vi "Imaging_Proc.vi"(5 "BioMAP file path":path=path "", 7 "Params.":variant, 8 "error in (no error)":errorcluster, 9 "Dynamic Params queue":refnum<queue>, 10 "Quit_UserEvent":refnum<user-event>, 11 "ControlQueueRef":variant) -> (0 "error out":errorcluster, 2 "Output":variant)   [LabVIEW 2013]
uses:
  Apps_static/ScanParams_SingleLine.ctl
  Files/BinaryHeader.ctl
  ControlDef/QueueRefs.ctl
  ControlDef/LaserCtrl_Method.ctl
  ControlDef/States-AToF.ctl
  <instrlib>/AnalogDiscSDKLv/VIs/DWF_CtrlQueue.ctl
  <instrlib>/AnalogDiscSDKLv/VIs/DWF_State.ctl
  <instrlib>/ESP300/Public/Data/ESP300_State.ctl
  <instrlib>/DG535/Command/DG535_States.ctl
  Hardware/BNC(QuantumComposers)/BNC_States.ctl
  Hardware/FemtoLaser(Legacy)/Laser_Status.ctl
  Hardware/DAQmx(Legacy)/DAQmx_Status.ctl
  ControlDef/Signal.ctl
  ProcessMethods/SignalAverager/ProcessStates.ctl
  Files/WriterState.ctl
  Files/Signal_Segment.ctl
  ControlDef/ProcessingMode.ctl
  Hardware/EPM2000(Legacy)/EPM2K_Status.ctl
  <instrlib>/AnalogDiscSDKLv/VIs/DWF_Signal.ctl
  ControlDef/SampleRateSelector.ctl
  DirectImaging_State.ctl
  Imaging_Params.ctl
  ProcessMethods/BioMapConversion/BioMAPWriterCoreParams.ctl
  <vilib>/Utility/miscctls.llb/LVRowAndColumnTypeDef.ctl
  <vilib>/picture/picture.llb/imagedata.ctl
  <userlib>/_OpenG.lib/comparison/comparison.llb/I32 Changed__ogtk.vi
  <vilib>/regexp/Match Regular Expression.xnode
  <instrlib>/ESP300/ESP300.lvlib
  <instrlib>/DG535/SRS_DG535_Lib.lvlib
  <userlib>/Utility/ErrorLog_lib.lvlib
  <instrlib>/AnalogDiscSDKLv/AnalogDiscSDKLv.lvlib
panel:
  in  "SaveImage":bool
  in  "Color Scheme":T1(ring)=enum."Rainbow"
  out "#SOL":i32
  out "#EOL":i32
  out "remaining lines":i32
  out "State":T2(ring)
  out "mzCali.":dbl[](array[numeric])
  out "Line#":i32
  in  "Cancel":bool
  in  "Close/Quit":bool
  in  "Peaks of Interest":string[][](table)=[["300", "300"], ["68", ".45"], ["92", ".45"], ["114", ".45"]]
  in  "conv. coeff.":sgl=6553.0
  out "# average":i32
  in  "Start":bool
  out "Intensity Graph":dbl[][](graph)
  in  "PeakOI #":i32
  out "MS (Raw)":cluster{"m/z_Array":dbl[], sgl[]}(graph)
  out "Iteration":i32
  out "Export File Path":path caption="Filename"
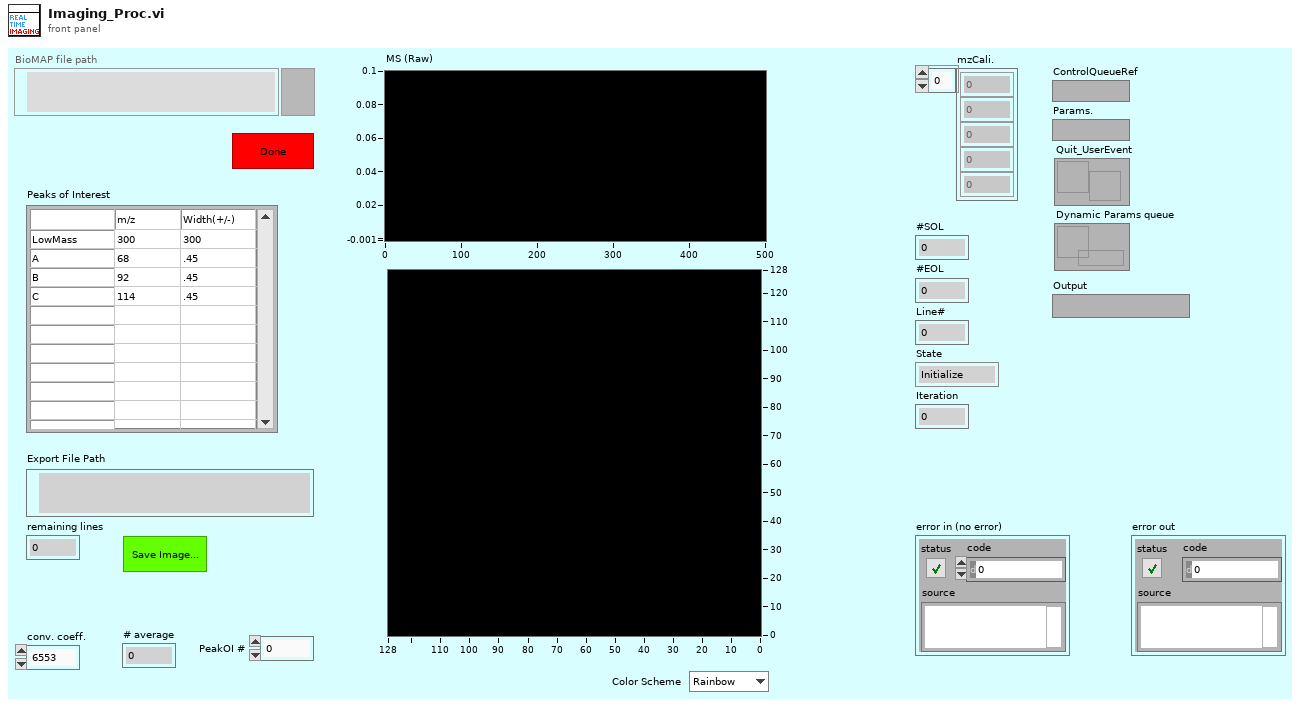
[diagram p1: front panel]
types:
  T1 = enum16{"Greyscale", "Rainbow", "Jet", "Rainbow_Wh", "Banded", "Seis", "InvertSeis", "Jaisnd", "TBD1"}
  T2 = enum16{"Initialize", "Open", "PrepScanParams", "WaitData", "Flush", "ScanResult", "CheckEndCondition", "Close", "Quit", "Refresh_Image", "Refresh_Profile", "Refresh_Spectra", "Refresh_RawSpectrum", "SaveMiddleFile"}
  T3 = enum8{"Enabled", "Disabled", "Disabled and Grayed Out"}
  T4 = typedef "QueueRefs.ctl" = cluster{"LaserCtrlMethod":T5, "Apps":refnum<queue>, "MainDAQCoreQueue":refnum<queue>, "Micos":refnum<queue>, "ESP300":refnum<queue>, "SMC100":refnum<queue>, "SRS DG535":refnum<queue>, "BNC":refnum<queue>, "SDG_ii":refnum<queue>, "NI-USB_DAQmx":refnum<queue>, "ProcCore_CtrlQueue":refnum<queue>, "WriterCtrl":refnum<queue>, "WriterSIG":refnum<queue>, "Feedback":refnum<queue>, "EPM2000":refnum<queue>, "InfoRef":refnum<vi>, "AppsLock":T6, "ProcCore_SignalQueue":refnum<queue>}
  T5 = typedef "LaserCtrl_Method.ctl" = enum16{"SRS_DG535", "BNC", "SDG_II"}
  T6 = typedef "Semaphore RefNum" = refnum<k1>
  T7 = typedef "ProcessStates.ctl" = enum16{"Initialize", "Normal", "Display", "Write2Buffer", "CalcMzArray", "StartSave", "StopSave", "ConfigChanged", "EndOfLine", "SetFilterParams", "SetGraphsEnable", "SetAcquisitionParams", "ChangeDisplayIncrement", "ChangeRepRate", "SetWriterRef", "Quit", "StartOfLine"}
  T8 = cluster{"Average":i32, "X (Img)":i32, "Y (Img)":i32, "Spectra":sgl[], "Depth":i32}
  T9 = typedef "BioMAPWriterCoreParams.ctl" = cluster{"File Header":T10, "mzCali.":dbl[], "m/z_Array":dbl[], "SampleRate":T11, "TrigDelay":dbl, "file refnum":refnum<file>, "file path":path, "PeakOI":cluster{"m/z":dbl, "Width(+/-)":dbl}[]}
  T10 = typedef "BinaryHeader.ctl" = cluster{"Start Position":dbl[], "StepWidth":dbl[], "Dimension":i32[], "SpecLength":i32}
  T11 = typedef "SampleRateSelector.ctl" = dbl
  T12 = typedef "Imaging_Params.ctl" = cluster{"File Header":T10, "ScanSpeed":dbl, "HighSpeed":dbl, "SampleRate":T11, "Rep.Rate (Hz)":dbl, "TrigDelay":dbl, "mzCali":dbl[], "KeepStill(ms)":u32, "SaveRaw":bool}
  T13 = typedef "DirectImaging_State.ctl" = cluster{"State":enum16{"Initialize", "Open", "PrepScanParams", "WaitData", "Flush", "ScanResult", "CheckEndCondition", "Close", "Quit", "Refresh_Image", "Refresh_Profile", "Refresh_Spectra", "Refresh_RawSpectrum", "SaveMiddleFile", "Save_Image"}, "Para.":variant}
  T14 = cluster{"Save?":bool, "File Header":T10, "Scan#":i32, "ControlRefs":T4, "HighSpeed":dbl, "ScanSpeed":dbl, "SampleRate":T11, "mzCali.":dbl[], "TrigDelay":dbl}
  T15 = typedef "LVRowAndColumnTypeDef.ctl" = cluster{"Row":i32, "Column":i32}
  T16 = cluster{"queue out":refnum<queue>, "queue out":refnum<queue>}
  T17 = typedef "Signal.ctl" = cluster{"Command":T7, "Params":variant}
  T18 = typedef "Signal_Segment.ctl" = cluster{"SampleRate":dbl, "TrigDelay":dbl, "SpecLength":dbl, "DAQ_Range":dbl, "Average#":i32, "Position":dbl[], "Spectrum":sgl[], "Calibr.":dbl[], "Pressure":dbl, "Desp_LaserEnergy":dbl, "PI_LaserEnergy":dbl, "Voltages Table":sgl[][], "ProcMode":T19, "Threshold":dbl, "Comment":string, "TickCount":dbl, "Time Stamp":timestamp}
  T19 = typedef "ProcessingMode.ctl" = enum16{"None", "Drop by Threshold", "TDC Simulate", "SetFilter"}
  T20 = enum16{"open", "replace", "create", "open or create", "replace or create", "replace or create with confirmation"}
  T21 = typedef "ScanParams_SingleLine.ctl" = cluster{"Start Position":dbl[], "End Position":dbl[], "HighSpeed":dbl, "ScanSpeed":dbl, "KeepStill(ms)":u32}
  T22 = cluster{"Dimension":u16, "SpecDepth":u16, "x dimension":u16, "y dimension":u16, "z dimension":u16}
  T23 = cluster{"Dimension 1":sgl, "Dimension 2":sgl, "Dimension 3":sgl, "Dimension 4":sgl, "Dimension 5":sgl, "Dimension 6":sgl, "Dimension 7":sgl, "Dimension 8":sgl}
  T24 = typedef "imagedata.ctl" = cluster{"image type":i32, "image depth":i32, "image":u8[], "mask":u8[], "colors":u32[], "Rectangle":cluster{"left":i16, "top":i16, "right":i16, "bottom":i16}}
  T25 = cluster{"Rows Per Strip":i32, "Photometric":i32, "Compression Type":i32}
  T26 = enum16{"Initialize", "Open", "PrepScanParams", "WaitData", "Flush", "ScanResult", "CheckEndCondition", "Close", "Quit", "Refresh_Image", "Refresh_Profile", "Refresh_Spectra", "Refresh_RawSpectrum", "SaveMiddleFile", "Save_Image"}
  T27 = typedef "IMAQ Image.ctl" = refnum<image>
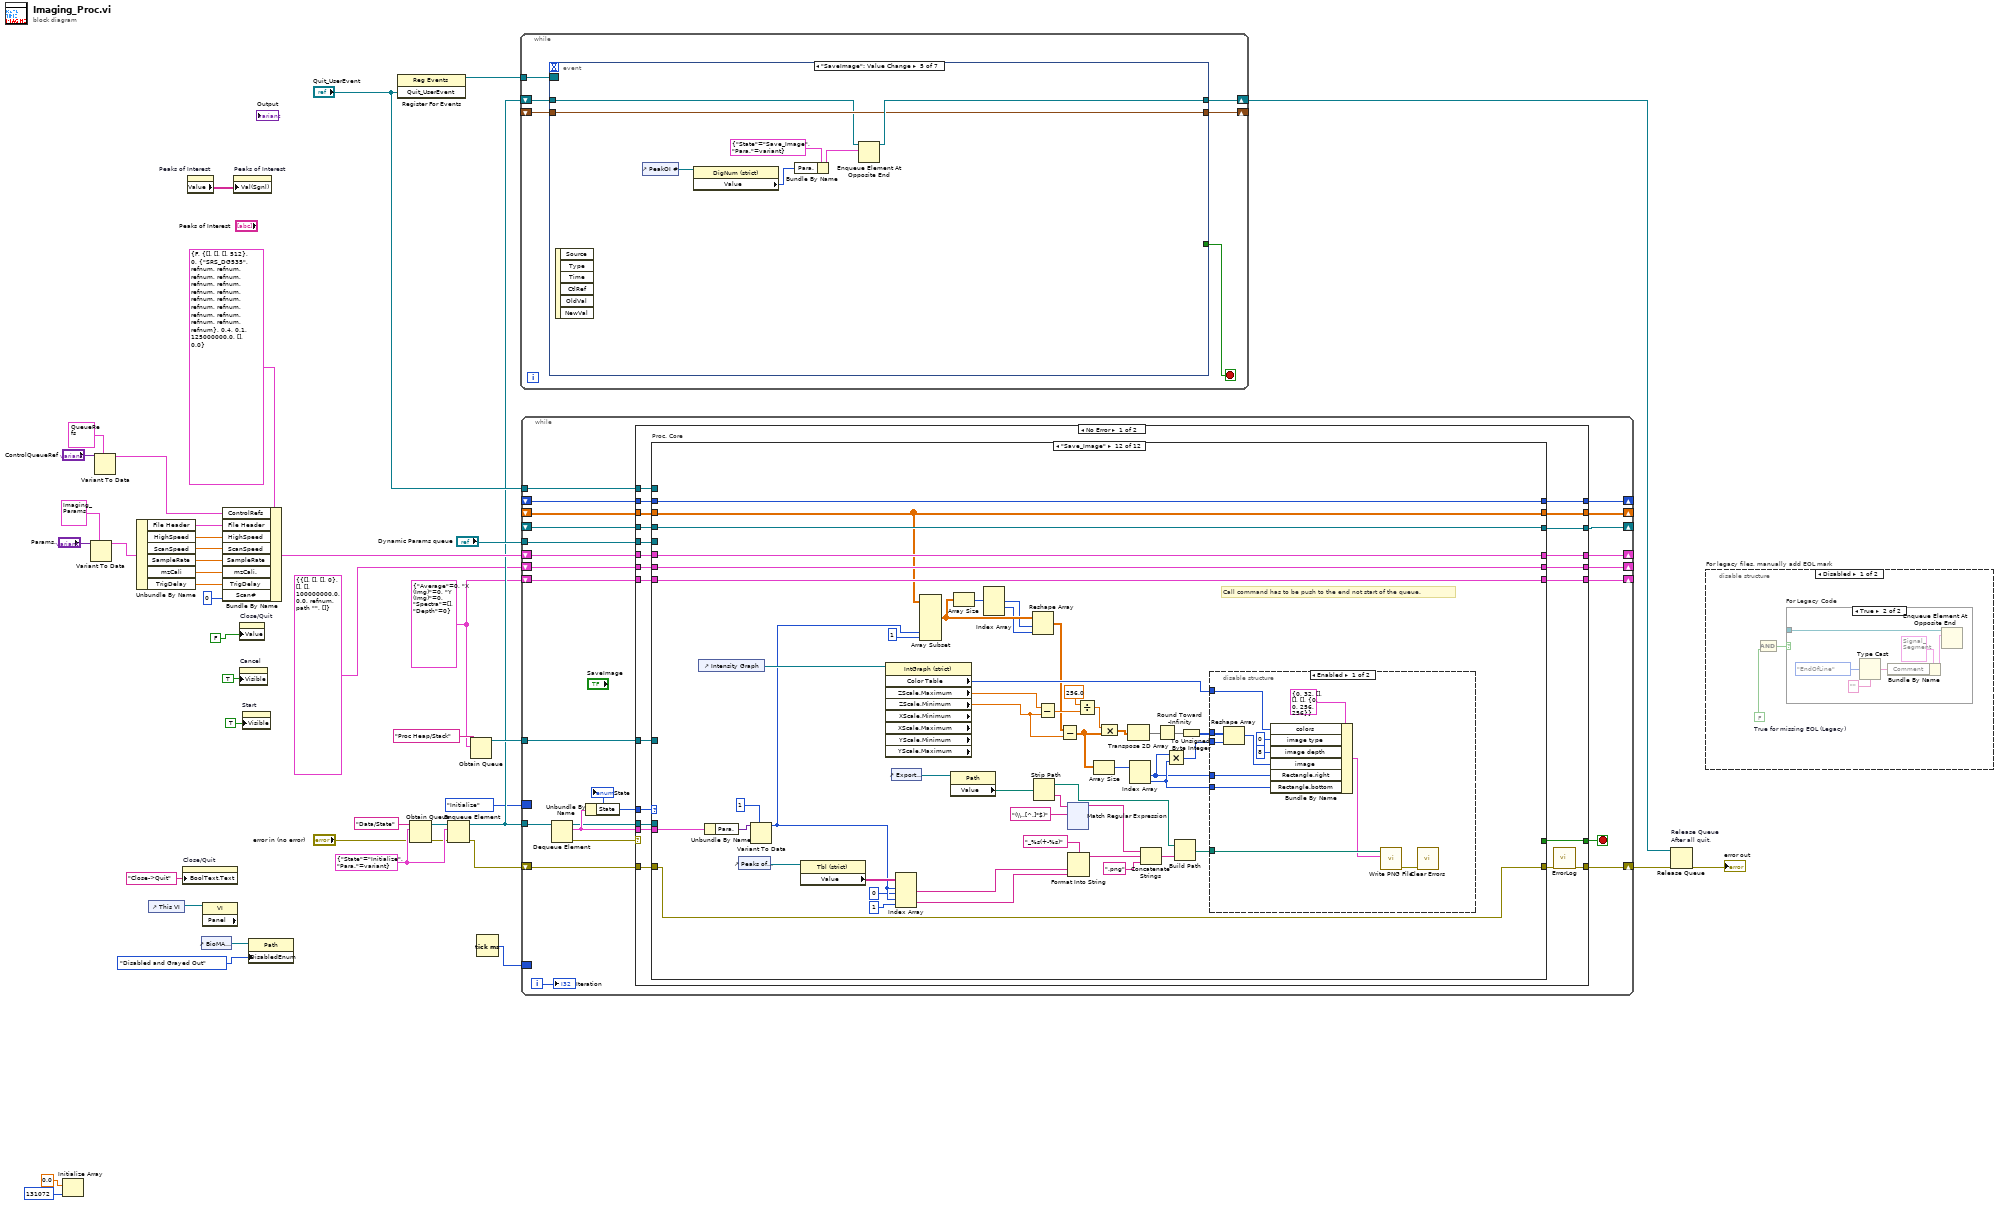
[diagram p0: block diagram]
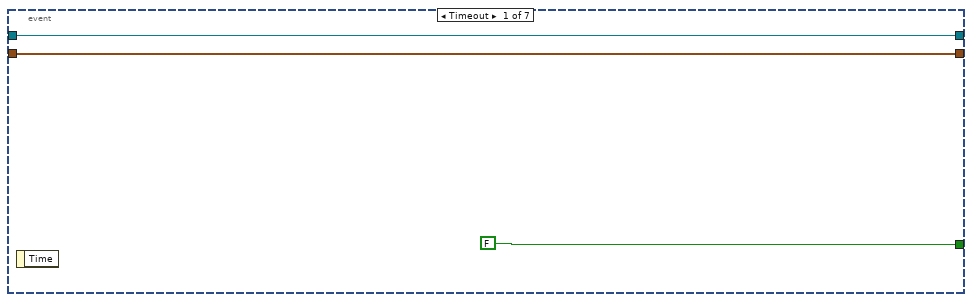
[diagram p4: hidden frame]
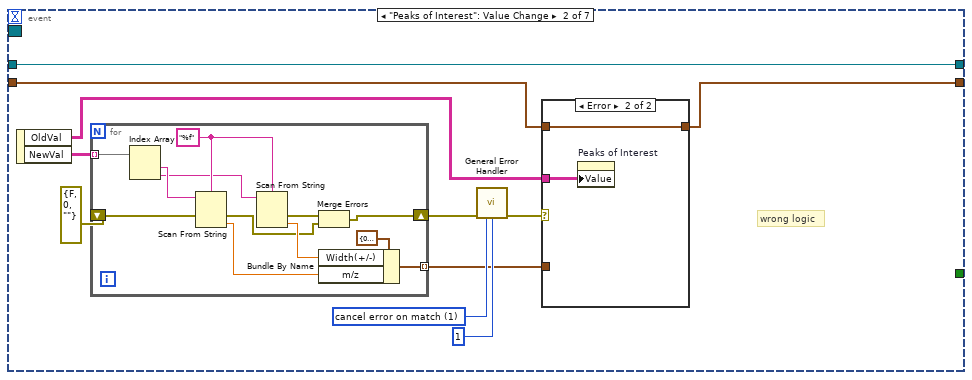
[diagram p5: hidden frame]
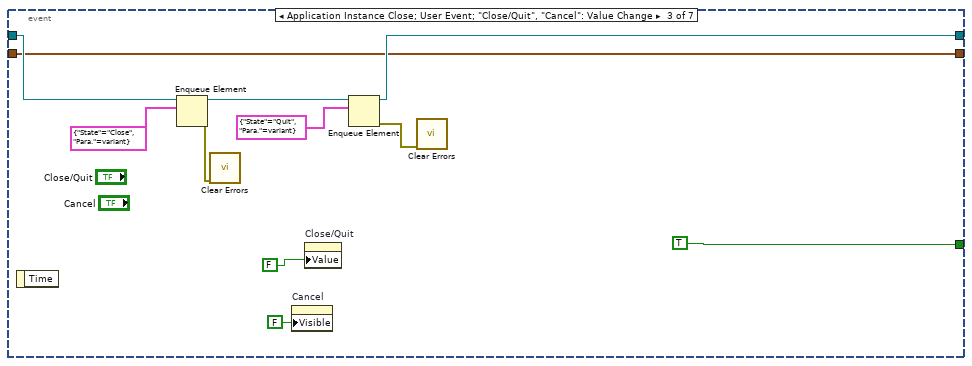
[diagram p7: hidden frame]
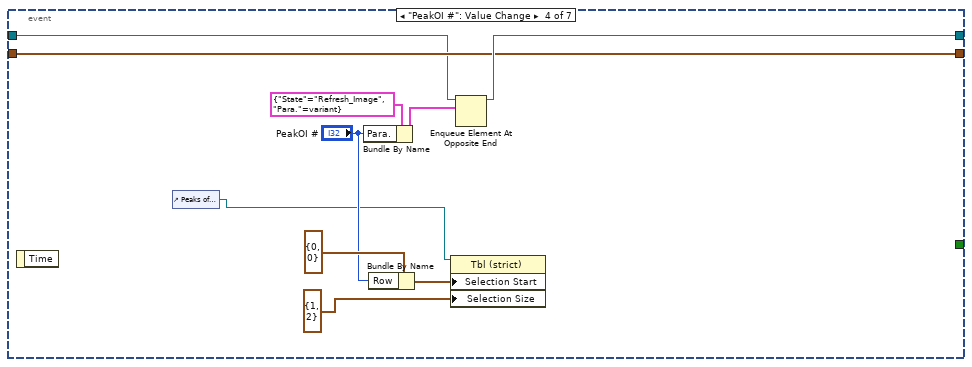
[diagram p8: hidden frame]
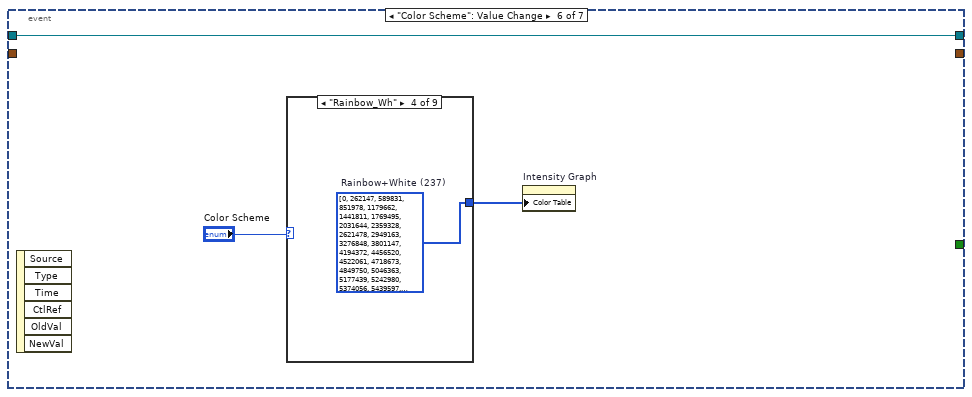
[diagram p9: hidden frame]
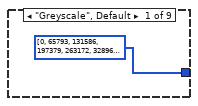
[diagram p10: hidden frame]
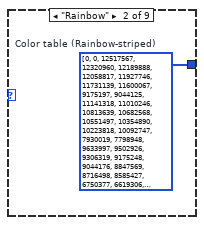
[diagram p11: hidden frame]
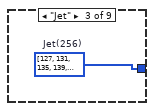
[diagram p12: hidden frame]
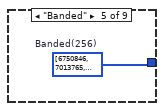
[diagram p13: hidden frame]
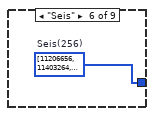
[diagram p14: hidden frame]
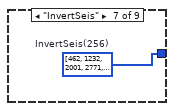
[diagram p15: hidden frame]
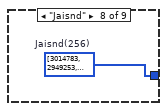
[diagram p16: hidden frame]
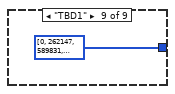
[diagram p17: hidden frame]
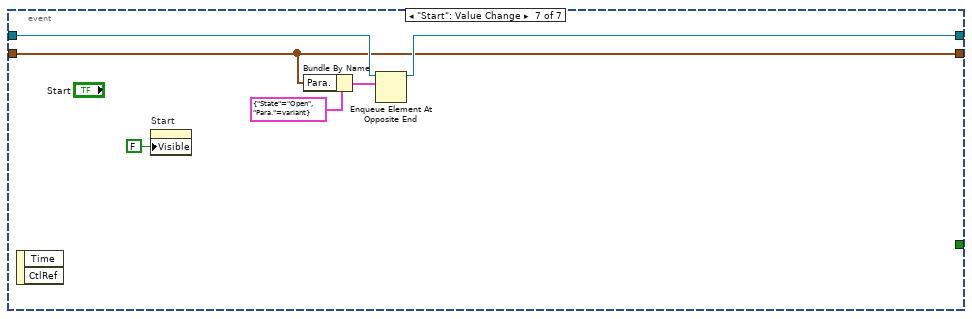
[diagram p18: hidden frame]
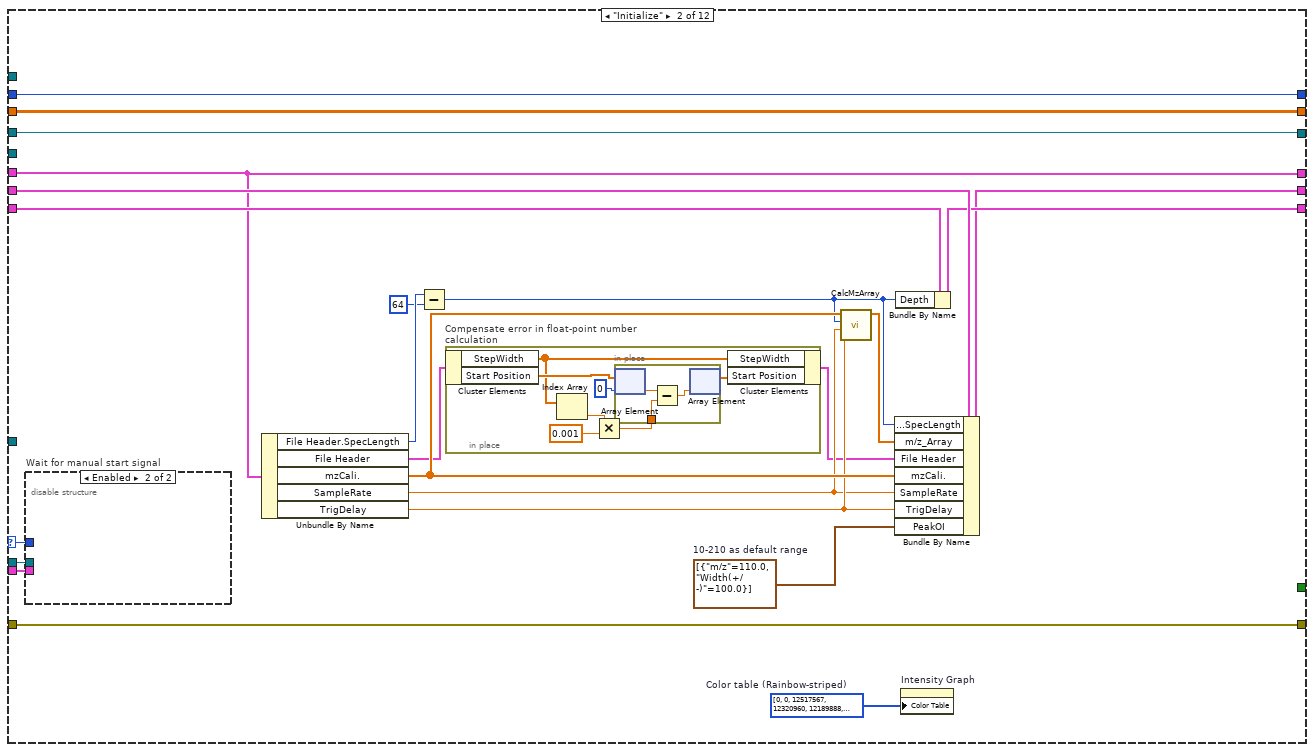
[diagram p20: hidden frame]
diagram:
  w22 = T8 {"Average"=0, "X (Img)"=0, "Y (Img)"=0, "Spectra"=[], "Depth"=0} ("output cluster")
  w34 = T13 {"State"=enum."Initialize", "Para."=variant}
  n1 = Initialize Array(sgl 0.0 ("element"), 131072 ("dimension size")) -> ()  [unwired: 1 out]
  n2 = Variant To Data(type=T12 {"File Header"={"Start Position"=[], "StepWidth"=[], "Dimension"=[], "SpecLength"=0}, "ScanSpeed"=0.0, "HighSpeed"=0.0, "SampleRate"=0.0, "Rep.Rate (Hz)"=0.0, "TrigDelay"=0.0, "mzCali"=[], "KeepStill(ms)"=0, "SaveRaw"=FALSE} ("BeamProfiling_Params"), Variant="Params.") -> (data=w29:T12)  [unwired: 1 in, 1 out]
  n3 = Variant To Data(type=T4 {"LaserCtrlMethod"=enum."SRS_DG535", "Apps"=refnum, "MainDAQCoreQueue"=refnum, "Micos"=refnum, "ESP300"=refnum, "SMC100"=refnum, "SRS DG535"=refnum, "BNC"=refnum, "SDG_ii"=refnum, "NI-USB_DAQmx"=refnum, "ProcCore_CtrlQueue"=refnum, "WriterCtrl"=refnum, "WriterSIG"=refnum, "Feedback"=refnum, "EPM2000"=refnum, "InfoRef"=refnum, "AppsLock"=refnum, "ProcCore_SignalQueue"=refnum} ("ControlRefs"), Variant="ControlQueueRef") -> (data=w8:T4)  [unwired: 1 in, 1 out]
  n4 = Unbundle By Name(w29) -> ("File Header"=w28:T10, "HighSpeed"=w27:dbl, "ScanSpeed"=w26:dbl, "SampleRate"=w24:T11, "mzCali"=w14:dbl[], "TrigDelay"=w13:dbl)
  n5 = control-ref of="This VI"() -> (w12:refnum<vi>)
  n6 = property on="Close/Quit" class="Bool (strict)"("BoolText.Text"="Close->Quit" ("Boolean Text.Text")) -> ()  [unwired: 2 in, 2 out]
  n7 = property on="Peaks of Interest" class="Tbl (strict)"() -> ("Value"=w2:string[][])  [unwired: 2 in, 2 out]
  n8 = control-ref of="BioMAP file path"() -> (w7:refnum<vi>)
  n9 = property class="VI" props=["Panel"](reference=w12) -> ()  [unwired: 1 in, 3 out]
  n10 = Bundle By Name(cluster=T14 {"Save?"=FALSE, "File Header"={"Start Position"=[], "StepWidth"=[], "Dimension"=[], "SpecLength"=512}, "Scan#"=0, "ControlRefs"={"LaserCtrlMethod"=enum."SRS_DG535", "Apps"=refnum, "MainDAQCoreQueue"=refnum, "Micos"=refnum, "ESP300"=refnum, "SMC100"=refnum, "SRS DG535"=refnum, "BNC"=refnum, "SDG_ii"=refnum, "NI-USB_DAQmx"=refnum, "ProcCore_CtrlQueue"=refnum, "WriterCtrl"=refnum, "WriterSIG"=refnum, "Feedback"=refnum, "EPM2000"=refnum, "InfoRef"=refnum, "AppsLock"=refnum, "ProcCore_SignalQueue"=refnum}, "HighSpeed"=0.4, "ScanSpeed"=0.1, "SampleRate"=125000000.0, "mzCali."=[], "TrigDelay"=0.0} ("output cluster"), "ControlRefs"=w8, "File Header"=w28, "HighSpeed"=w27, "ScanSpeed"=w26, "SampleRate"=w24, "mzCali."=w14, "TrigDelay"=w13, "Scan#"=0) -> (w38:T14)
  n11 = property on="Peaks of Interest" class="Tbl (strict)"("Val(Sgnl)"=w2) -> ()  [unwired: 2 in, 2 out]
  n12 = property on="Close/Quit" class="Bool (strict)"("Value"=FALSE) -> ()  [unwired: 2 in, 2 out]
  n13 = property on="Cancel" class="Bool"("Visible"=TRUE) -> ()  [unwired: 2 in, 2 out]
  n14 = property on="Start" class="Bool"("Visible"=TRUE) -> ()  [unwired: 2 in, 2 out]
  n15 = property class="Path"(reference=w7, "DisabledEnum"=T3."Disabled and Grayed Out" ("Disabled")) -> ()  [unwired: 1 in, 2 out]
  n16 = register-events("Quit_UserEvent") -> (reference out=w39:refnum<event-registration>)  [unwired: 2 in, 1 out]
  n17 = Obtain Queue(name (unnamed)="Data/State", element data type=w34, error in (no error)="error in (no error)") -> (queue out=w35:refnum<queue>, error out=w33:errorcluster)  [unwired: 2 in, 1 out]
  n18 = Enqueue Element(queue=w35, element=w34, error in (no error)=w33) -> (queue out=w31:refnum<queue>, error out=w23:errorcluster)  [unwired: 1 in, 1 out]
  n19 = Obtain Queue(name (unnamed)="Proc Heap/Stack", element data type=w22) -> (queue out=w44:refnum<queue>)  [unwired: 3 in, 2 out]
  n20 = Tick Count (ms)() -> (millisecond timer value=w21:u32)
  n21 = while {
    tunnel: w39 -> [w48]
    shift-right: [w47] -> w15
    shift-left: w31 -> [w50]
    shift-right: [w46] -> _
    shift-left: _ -> [w45]
    stop <- w49 stop-if-true
    n22 = event shown="[4] \"SaveImage\": Value Change" {
      selector: w48 -> [_ _ _ _ _ _ _]
      dyn-events: _ -> [_ _ _ _ _ _ _]
      timeout: _ -> [_ _ _ _ _ _ _]
      tunnel: w50 -> [w52 w62 w87 w96 w103 w110 w125]
      tunnel: [FALSE _ TRUE _ _ _ _] -> w49
      tunnel: [w52 w62 w83 w98 w105 w110 w123] -> w47
      tunnel: [w51 w56 w82 w97 w104 _ w121] -> w46
      tunnel: w45 -> [w51 w54 w82 w97 w104 _ w121]
      event Timeout {
        n23 = event-data() -> ()  [unwired: 1 in, 1 out]
      }
      event "Peaks of Interest": Value Change {
        w57 = 1 items=["no exception", "cancel error on match", "set error on match"] ("[exception action] (none:0)")
        # "wrong logic"
        n24 = event-data() -> ("OldVal"=w63:string[][], "NewVal"=w64:string[][])  [unwired: 1 in]
        n25 = for {
          tunnel: w64 -> [w76] mode=indexing
          shift-right: [w68] -> w58
          shift-left: errorcluster {"status"=FALSE, "code"=0, "source"=""} ("error IO") -> [w70]
          tunnel: [w69] -> w55 mode=indexing
          w75 = "%f" ("format string")
          n26 = Index Array(array=w76) -> (element #1=w66:string, element #2=w65:string)  [unwired: 2 in]
          n27 = Scan From String(format string=w75, input string=w66, error in=w70) -> (error out=w67:errorcluster, output 1=w72:dbl)  [unwired: 2 in, 2 out]
          n28 = Scan From String(format string=w75, input string=w65) -> (error out=w71:errorcluster, output 1=w73:dbl)  [unwired: 3 in, 2 out]
          n29 = Merge Errors(w71, w67) -> (w68:errorcluster)
          n30 = Bundle By Name(cluster=cluster{"m/z":dbl, "Width(+/-)":dbl} {"m/z"=0.0, "Width(+/-)"=0.0} ("Peak-Of-Interest"), "Width(+/-)"=w73, "m/z"=w72) -> (w69:cluster{"m/z":dbl, "Width(+/-)":dbl})
        }
        n31 = call <vilib>:"General Error Handler.vi"("error in (no error)"=w58, "[exception action] (none:0)"=w57, "[exception code]"=1) -> ("error out"=w59:errorcluster)  [unwired: 8 in, 4 out]
        n32 = case shown="Error" w59 {
          tunnel: w63 -> [_ w79]
          tunnel: [w77 w78] -> w56
          tunnel: w55 -> [w77 _]
          tunnel: w54 -> [_ w78]
          frame No Error {
          }
          frame Error {
            n33 = property on="Peaks of Interest" class="Tbl (strict)"("Value"=w79) -> ()  [unwired: 2 in, 2 out]
          }
        }
      }
      event Application Instance Close; User Event; "Close/Quit", "Cancel": Value Change {
        n34 = event-data() -> ()  [unwired: 1 in, 1 out]
        n35 = Enqueue Element(queue=w87, element=T13 {"State"=enum."Close", "Para."=variant}) -> (queue out=w88:refnum<queue>, error out=w86:errorcluster)  [unwired: 2 in, 1 out]
        n36 = call <vilib>:"Clear Errors.vi"("error in (no error)"=w86) -> ()  [unwired: 6 in, 1 out]
        n37 = property on="Cancel" class="Bool"("Visible"=FALSE) -> ()  [unwired: 2 in, 2 out]
        n38 = property on="Close/Quit" class="Bool (strict)"("Value"=FALSE) -> ()  [unwired: 2 in, 2 out]
        n39 = Enqueue Element(queue=w88, element=T13 {"State"=enum."Quit", "Para."=variant}) -> (queue out=w83:refnum<queue>, error out=w89:errorcluster)  [unwired: 2 in, 1 out]
        n40 = call <vilib>:"Clear Errors.vi"("error in (no error)"=w89) -> ()  [unwired: 6 in, 1 out]
      }
      event "PeakOI #": Value Change {
        n41 = event-data() -> ()  [unwired: 1 in, 1 out]
        n42 = control-ref of="Peaks of Interest"() -> (w91:refnum<vi>)
        n43 = Bundle By Name(cluster=T13 {"State"=enum."Refresh_Image", "Para."=variant} ("element"), "Para."="PeakOI #") -> (w99:T13)
        n44 = Bundle By Name(cluster=T15 {"Row"=0, "Column"=0} ("Selection Start"), "Row"="PeakOI #") -> (w94:T15)
        n45 = property on="Property Node" class="Tbl (strict)"(reference=w91, "Selection Start"=w94, "Selection Size"=T15 {"Row"=1, "Column"=2}) -> ()  [unwired: 1 in, 2 out]
        n46 = Enqueue Element At Opposite End(queue=w96, element=w99) -> (queue out=w98:refnum<queue>)  [unwired: 2 in, 2 out]
      }
      event "SaveImage": Value Change {
        n47 = event-data() -> ()  [unwired: 1 in, 6 out]
        n48 = control-ref of="PeakOI #"() -> (w102:refnum<vi>)
        n49 = property class="DigNum (strict)"(reference=w102) -> ("Value"=w101:i32)  [unwired: 1 in, 2 out]
        n50 = Bundle By Name(cluster=T13 {"State"=enum."Save_Image", "Para."=variant} ("element"), "Para."=w101) -> (w106:T13)
        n51 = Enqueue Element At Opposite End(queue=w103, element=w106) -> (queue out=w105:refnum<queue>)  [unwired: 2 in, 2 out]
      }
      event "Color Scheme": Value Change {
        n52 = event-data() -> ()  [unwired: 1 in, 6 out]
        n53 = case shown="\"Rainbow_Wh\"" "Color Scheme" {
          tunnel: [u32[] [0, 65793, 131586, 197379, 263172, 328965, 394758, 460551, 526344, 592137, 657930, 723723, 789516, 855309, 921102, 986895, 1052688, 1118481, 1184274, 1250067, 1315860, 1381653, 1447446, 1513239, 1579032, 1644825, 1710618, 1776411, 1842204, 1907997, 1973790, 2039583, 2105376, 2171169, 2236962, 2302755, 2368548, 2434341, 2500134, 2565927, 2631720, 2697513, 2763306, 2829099, 2894892, 2960685, 3026478, 3092271, 3158064, 3223857, 3289650, 3355443, 3421236, 3487029, 3552822, 3618615, 3684408, 3750201, 3815994, 3881787, 3947580, 4013373, 4079166, 4144959, 4210752, 4276545, 4342338, 4408131, 4473924, 4539717, 4605510, 4671303, 4737096, 4802889, 4868682, 4934475, 5000268, 5066061, 5131854, 5197647, 5263440, 5329233, 5395026, 5460819, 5526612, 5592405, 5658198, 5723991, 5789784, 5855577, 5921370, 5987163, 6052956, 6118749, 6184542, 6250335, 6316128, 6381921, 6447714, 6513507, 6579300, 6645093, 6710886, 6776679, 6842472, 6908265, 6974058, 7039851, 7105644, 7171437, 7237230, 7303023, 7368816, 7434609, 7500402, 7566195, 7631988, 7697781, 7763574, 7829367, 7895160, 7960953, 8026746, 8092539, 8158332, 8224125, 8289918, 8355711, 8421504, 8487297, 8553090, 8618883, 8684676, 8750469, 8816262, 8882055, 8947848, 9013641, 9079434, 9145227, 9211020, 9276813, 9342606, 9408399, 9474192, 9539985, 9605778, 9671571, 9737364, 9803157, 9868950, 9934743, 10000536, 10066329, 10132122, 10197915, 10263708, 10329501, 10395294, 10461087, 10526880, 10592673, 10658466, 10724259, 10790052, 10855845, 10921638, 10987431, 11053224, 11119017, 11184810, 11250603, 11316396, 11382189, 11447982, 11513775, 11579568, 11645361, 11711154, 11776947, 11842740, 11908533, 11974326, 12040119, 12105912, 12171705, 12237498, 12303291, 12369084, 12434877, 12500670, 12566463, 12632256, 12698049, 12763842, 12829635, 12895428, 12961221, 13027014, 13092807, 13158600, 13224393, 13290186, 13355979, 13421772, 13487565, 13553358, 13619151, 13684944, 13750737, 13816530, 13882323, 13948116, 14013909, 14079702, 14145495, 14211288, 14277081, 14342874, 14408667, 14474460, 14540253, 14606046, 14671839, 14737632, 14803425, 14869218, 14935011, 15000804, 15066597, 15132390, 15198183, 15263976, 15329769, 15395562, 15461355, 15527148, 15592941, 15658734, 15724527, 15790320, 15856113, 15921906, 15987699, 16053492, 16119285, 16185078, 16250871, 16316664, 16382457, 16448250, 16514043, 16579836, 16645629, 16711422, 16777215] ("Array") w112 w113 w114 w115 w116 w117 w118 u32[] [0, 262147, 589831, 851978, 1179662, 1441811, 1769495, 2031644, 2359328, 2621478, 2949163, 3276848, 3801147, 4194372, 4456520, 4522061, 4718673, 4849750, 5046363, 5177439, 5242980, 5374056, 5439597, 5505142, 5636218, 5767300, 5636232, 5701773, 5701777, 5701782, 5570714, 5505183, 5505187, 5505192, 5177521, 5111990, 5046458, 4980927, 4587720, 4456652, 4325585, 3932374, 3801306, 3604703, 3014888, 2818284, 2621681, 2359541, 2162938, 1638655, 1048831, 786687, 262399, 255, 1279, 4351, 5631, 6655, 7679, 9983, 11007, 12031, 13311, 16383, 17407, 18687, 21759, 23039, 24063, 25087, 27391, 28415, 29439, 30719, 32767, 34815, 36095, 39167, 40447, 41471, 42495, 44799, 45823, 46847, 48127, 50175, 51199, 55551, 56575, 57855, 58879, 59903, 62207, 63231, 64255, 65535, 65526, 65522, 65518, 65505, 65496, 65492, 65483, 65479, 65475, 65471, 65467, 65458, 65454, 65450, 65437, 65432, 65424, 65415, 65411, 65407, 65403, 65394, 65390, 65386, 65382, 65369, 65364, 65360, 65356, 65343, 65339, 65335, 65326, 65322, 65318, 65305, 65301, 65296, 65292, 65288, 65280, 589568, 851712, 1441536, 1703680, 1965824, 2817792, 3079936, 3407616, 3669760, 4194048, 4456192, 4783872, 5046016, 5897984, 6160128, 6422272, 7274240, 7536384, 7864064, 8126208, 8650496, 8912640, 9240320, 9502464, 10092288, 10616576, 10878720, 11730688, 11992832, 12320512, 12582656, 13106944, 13369088, 13696768, 13958912, 14548736, 14810880, 15924992, 16187136, 16449280, 16776960, 16775680, 16773632, 16772608, 16771328, 16770304, 16768256, 16766976, 16765952, 16762624, 16760576, 16759552, 16757248, 16756224, 16755200, 16753920, 16752896, 16750848, 16749568, 16748544, 16745216, 16744192, 16742144, 16739840, 16738816, 16737792, 16736512, 16734464, 16733440, 16732160, 16731136, 16727808, 16726784, 16725760, 16724736, 16721408, 16720384, 16719104, 16717056, 16716032, 16714752, 16711680, 16711680, 16711680, 16711680, 16711680, 16711680, 16711680, 16711680, 16711680, 16711680, 16711680, 16711680, 16711680, 16711680, 16711680, 16711680, 16711680, 16711680, 15527148, 15592941, 15658734, 15724527, 15790320, 15856113, 15921906, 15987699, 16053492, 16119285, 16185078, 16250871, 16316664, 16382457, 16448250, 16514043, 16579836, 16645629, 16711422, 16777215] ("appended array")] -> w108
          frame "Greyscale", Default {
          }
          frame "Rainbow" {
            w112 = u32[] [0, 0, 12517567, 12320960, 12189888, 12058817, 11927746, 11731139, 11600067, 9175197, 9044125, 11141318, 11010246, 10813639, 10682568, 10551497, 10354890, 10223818, 10092747, 7930019, 7798948, 9633997, 9502926, 9306319, 9175248, 9044176, 8847569, 8716498, 8585427, 6750377, 6619306, 8126677, 7995606, 7798999, 7667927, 7536856, 7340249, 7209178, 7078106, 5505199, 5374128, 6619357, 6488285, 6291678, 6160607, 6029536, 5832929, 5701857, 5570786, 4325557, 4194486, 5112036, 4980965, 4784358, 4653287, 4522215, 4325608, 4194537, 4063466, 3080380, 3014844, 3604716, 3408109, 3277038, 3277038, 3145966, 3014895, 2818288, 2687217, 2556145, 1900738, 1769666, 2097396, 1900789, 1769717, 1638646, 1507575, 1310968, 1179896, 1048825, 721096, 590024, 590075, 393468, 262397, 131326, 255, 1791, 3327, 4863, 5068, 6348, 9471, 11007, 12543, 14079, 15615, 17151, 18687, 20223, 17612, 18636, 25087, 26623, 28159, 29695, 31231, 32767, 34303, 35839, 29900, 31180, 40447, 41983, 43775, 45311, 46847, 48383, 49919, 51455, 42444, 43724, 56063, 57599, 59135, 60671, 62207, 63743, 65535, 65528, 52418, 52413, 65510, 65504, 65498, 65492, 65486, 65480, 65474, 65468, 52369, 52364, 65449, 65443, 65437, 65431, 65425, 65419, 65413, 65407, 52321, 52316, 65389, 65383, 65377, 65371, 65364, 65358, 65352, 65346, 52272, 52267, 65328, 65322, 65316, 65310, 65304, 65298, 65292, 65286, 52224, 314368, 851712, 1244928, 1638144, 2031360, 2424576, 2817792, 3211008, 3604224, 3197952, 3525632, 4783872, 5177088, 5635840, 6029056, 6422272, 6815488, 7208704, 7601920, 6409216, 6736896, 6736896, 8781568, 9174784, 9568000, 9961216, 10354432, 10747648, 11206400, 11599616, 9554944, 9882624, 12779264, 13172480, 13565696, 13958912, 14352128, 14745344, 15138560, 15531776, 12766208, 13093888, 16776960, 16775170, 16773637, 16771847, 16770314, 16768780, 16766991, 16765457, 13411088, 13409810, 16760601, 16758812, 16757278, 16755745, 16753955, 16752422, 16750888, 16749099, 13398052, 13396774, 16744243, 16742704, 16741166, 16739884, 16738345, 16736807, 16735269, 16733730, 13385753, 13384728, 16729371, 16727833, 16726295, 16725012, 16723474, 16721936, 16720397, 16718859, 13373959, 13372677, 16714500, 16712962, 16777215]  # Color table (Rainbow-striped)
          }
          frame "Jet" {
            w113 = u32[] [127, 131, 135, 139, 143, 147, 151, 155, 159, 163, 167, 171, 175, 179, 183, 187, 191, 195, 199, 203, 207, 211, 215, 219, 223, 227, 231, 235, 239, 243, 247, 251, 255, 1279, 2303, 3327, 4351, 5375, 6399, 7423, 8447, 9471, 10495, 11519, 12543, 13567, 14591, 15615, 16639, 17663, 18687, 19711, 20735, 21759, 22783, 23807, 24831, 25855, 26879, 27903, 28927, 29951, 30975, 31999, 33023, 34047, 35071, 36095, 37119, 38143, 39167, 40191, 41215, 42239, 43263, 44287, 45311, 46335, 47359, 48383, 49407, 50431, 51455, 52479, 53503, 54527, 55551, 56575, 57599, 58623, 59647, 60671, 61695, 62719, 63743, 64767, 131069, 393209, 655349, 917489, 1179629, 1441769, 1703909, 1966049, 2228189, 2490329, 2752469, 3014609, 3276749, 3538889, 3801029, 4063169, 4325309, 4587449, 4849589, 5111729, 5373869, 5636009, 5898149, 6160289, 6422429, 6684569, 6946709, 7208849, 7470989, 7733129, 7995269, 8257409, 8519549, 8781689, 9043829, 9305969, 9568109, 9830249, 10092389, 10354529, 10616669, 10878809, 11140949, 11403089, 11665229, 11927369, 12189509, 12451649, 12713789, 12975929, 13238069, 13500209, 13762349, 14024489, 14286629, 14548769, 14810909, 15073049, 15335189, 15597329, 15859469, 16121609, 16383749, 16645889, 16776192, 16775168, 16774144, 16773120, 16772096, 16771072, 16770048, 16769024, 16768000, 16766976, 16765952, 16764928, 16763904, 16762880, 16761856, 16760832, 16759808, 16758784, 16757760, 16756736, 16755712, 16754688, 16753664, 16752640, 16751616, 16750592, 16749568, 16748544, 16747520, 16746496, 16745472, 16744448, 16743424, 16742400, 16741376, 16740352, 16739328, 16738304, 16737280, 16736256, 16735232, 16734208, 16733184, 16732160, 16731136, 16730112, 16729088, 16728064, 16727040, 16726016, 16724992, 16723968, 16722944, 16721920, 16720896, 16719872, 16718848, 16717824, 16716800, 16715776, 16714752, 16713728, 16712704, 16711680, 16449536, 16187392, 15925248, 15663104, 15400960, 15138816, 14876672, 14614528, 14352384, 14090240, 13828096, 13565952, 13303808, 13041664, 12779520, 12517376, 12255232, 11993088, 11730944, 11468800, 11206656, 10944512, 10682368, 10420224, 10158080, 9895936, 9633792, 9371648, 9109504, 8847360, 8585216, 8323072]  # Jet(256)
          }
          frame "Rainbow_Wh" {
            w114 = u32[] [0, 262147, 589831, 851978, 1179662, 1441811, 1769495, 2031644, 2359328, 2621478, 2949163, 3276848, 3801147, 4194372, 4456520, 4522061, 4718673, 4849750, 5046363, 5177439, 5242980, 5374056, 5439597, 5505142, 5636218, 5767300, 5636232, 5701773, 5701777, 5701782, 5570714, 5505183, 5505187, 5505192, 5177521, 5111990, 5046458, 4980927, 4587720, 4456652, 4325585, 3932374, 3801306, 3604703, 3014888, 2818284, 2621681, 2359541, 2162938, 1638655, 1048831, 786687, 262399, 255, 1279, 4351, 5631, 6655, 7679, 9983, 11007, 12031, 13311, 16383, 17407, 18687, 21759, 23039, 24063, 25087, 27391, 28415, 29439, 30719, 32767, 34815, 36095, 39167, 40447, 41471, 42495, 44799, 45823, 46847, 48127, 50175, 51199, 55551, 56575, 57855, 58879, 59903, 62207, 63231, 64255, 65535, 65526, 65522, 65518, 65505, 65496, 65492, 65483, 65479, 65475, 65471, 65467, 65458, 65454, 65450, 65437, 65432, 65424, 65415, 65411, 65407, 65403, 65394, 65390, 65386, 65382, 65369, 65364, 65360, 65356, 65343, 65339, 65335, 65326, 65322, 65318, 65305, 65301, 65296, 65292, 65288, 65280, 589568, 851712, 1441536, 1703680, 1965824, 2817792, 3079936, 3407616, 3669760, 4194048, 4456192, 4783872, 5046016, 5897984, 6160128, 6422272, 7274240, 7536384, 7864064, 8126208, 8650496, 8912640, 9240320, 9502464, 10092288, 10616576, 10878720, 11730688, 11992832, 12320512, 12582656, 13106944, 13369088, 13696768, 13958912, 14548736, 14810880, 15924992, 16187136, 16449280, 16776960, 16775680, 16773632, 16772608, 16771328, 16770304, 16768256, 16766976, 16765952, 16762624, 16760576, 16759552, 16757248, 16756224, 16755200, 16753920, 16752896, 16750848, 16749568, 16748544, 16745216, 16744192, 16742144, 16739840, 16738816, 16737792, 16736512, 16734464, 16733440, 16732160, 16731136, 16727808, 16726784, 16725760, 16724736, 16721408, 16720384, 16719104, 16717056, 16716032, 16714752, 16711680, 16711680, 16711680, 16711680, 16711680, 16711680, 16711680, 16711680, 16711680, 16711680, 16711680, 16711680, 16711680, 16711680, 16711680, 16711680, 16711680, 16711680, 16777215, 16777215, 16777215, 16777215, 16777215, 16777215, 16777215, 16777215, 16777215, 16777215, 16777215, 16777215, 16777215, 16777215, 16777215, 16777215, 16777215, 16777215, 16777215, 16777215]  # Rainbow+White (237)
          }
          frame "Banded" {
            w115 = u32[] [6750846, 7013765, 7211659, 7409807, 7476371, 7411604, 7214997, 7017621, 6754453, 6490776, 6358685, 6226596, 6226092, 6226101, 6226109, 6227140, 6293961, 6296012, 6297806, 6233806, 5906635, 5512904, 4922053, 4199363, 3542212, 2950855, 2425550, 2031830, 1638622, 1376741, 1246954, 1314285, 1447407, 1975278, 2305771, 2372838, 2242272, 1783259, 1323992, 799448, 340956, 79842, 15849, 17905, 151543, 481786, 1009148, 1667324, 2193914, 2457333, 2523375, 2260968, 1801698, 1276895, 752607, 360418, 99816, 36335, 38390, 237307, 632574, 1158654, 1815550, 2275323, 2537717, 2471662, 2208487, 1683426, 1158879, 634847, 308451, 48362, 50673, 52728, 316924, 777214, 1302782, 1893373, 2352122, 2548212, 2481645, 2087398, 1628129, 1038303, 580576, 254949, 60394, 62189, 129520, 392688, 851694, 1441515, 2031078, 2423264, 2552791, 2419661, 2024898, 1499321, 974770, 516526, 190124, 60844, 62635, 129707, 458153, 982695, 1572516, 2161825, 2488475, 2552211, 2353800, 1893501, 1368177, 843623, 451166, 124759, 61010, 62797, 195401, 589383, 1113670, 1703494, 2227014, 2553410, 2551868, 2287665, 1827364, 1302294, 974603, 1040900, 1239041, 1699840, 2291200, 3013379, 3866121, 4783634, 5635611, 6355746, 6878502, 7073317, 7071521, 7004697, 6938385, 7069705, 7398403, 7858688, 8515840, 9172992, 9894916, 10550795, 11140627, 11599132, 11926051, 12055590, 11988261, 11855391, 11723032, 11788047, 11984904, 12510467, 13101824, 13759232, 14416129, 15006981, 15400460, 15728149, 15858974, 15857956, 15659558, 15395620, 15065886, 14736150, 14669582, 14800391, 15128322, 15587840, 16047616, 16441345, 16637958, 16703246, 16702743, 16570656, 16307237, 15846438, 15385379, 14924316, 14660116, 14658828, 14854661, 15182337, 15641344, 16100352, 16493826, 16690440, 16690192, 16690201, 16492833, 16163878, 15703078, 15242018, 14846235, 14647058, 14645003, 14840068, 15232513, 15690496, 16083200, 16410371, 16541193, 16541202, 16410139, 16213282, 15818789, 15292709, 14831136, 14434840, 14169616, 14166537, 14360579, 14686208, 15077888, 15404288, 15600132, 15665675, 15536665, 15342119, 15015986, 14558008, 14033211, 13507643, 13047097, 12848439, 12781367, 12911162, 13107263, 13303877, 13500748, 13501524, 13371996, 13177188, 12851050, 12393581, 11869549, 11278955, 10753384, 10293092, 9963875, 9765987, 9765220, 9764967, 9699434, 9634157, 9372526, 9111662, 8719469, 8261738]  # Banded(256)
          }
          frame "Seis" {
            w116 = u32[] [11206656, 11403264, 11599872, 11796480, 11993088, 12189696, 12386304, 12582912, 12779520, 12976128, 13172736, 13369344, 13565952, 13762560, 13959168, 14155776, 14352384, 14548992, 14745600, 14942208, 15138816, 15335424, 15532032, 15728640, 15925248, 16121856, 16318464, 16515072, 16711680, 16712448, 16713216, 16713984, 16714752, 16715520, 16716288, 16717056, 16717824, 16718592, 16719360, 16720128, 16720896, 16721664, 16722432, 16723200, 16723968, 16724736, 16725504, 16726272, 16727040, 16727808, 16728576, 16729344, 16730112, 16730880, 16731648, 16732416, 16733184, 16733952, 16734720, 16735488, 16736256, 16737024, 16737792, 16738560, 16739328, 16740096, 16740864, 16741632, 16742400, 16743168, 16743936, 16744448, 16745216, 16745984, 16746752, 16747520, 16748288, 16749056, 16749824, 16750592, 16751360, 16752128, 16752896, 16753664, 16754432, 16755200, 16755968, 16756736, 16757504, 16758272, 16759040, 16759808, 16760576, 16761344, 16762112, 16762880, 16763648, 16764416, 16765184, 16765952, 16766720, 16767488, 16768256, 16769024, 16769792, 16770560, 16771328, 16772096, 16772864, 16773632, 16774400, 16775168, 16775936, 16776704, 16776960, 16776960, 16776960, 16776960, 16776960, 16776960, 16776960, 16776960, 16776960, 16776960, 16776960, 16776960, 16776960, 16776960, 16776960, 16776960, 16776960, 16776960, 16776960, 16776960, 16776960, 16776960, 16776960, 16776960, 16776960, 16776960, 16776960, 16776960, 16645888, 16252673, 15924994, 15531779, 15138565, 14745350, 14352135, 14024456, 13631241, 13238026, 12844811, 12451596, 12123917, 11730702, 11337487, 10944272, 10551057, 10223378, 9830163, 9436948, 9043733, 8650518, 8322840, 7929625, 7536410, 7143195, 6749980, 6422301, 6029086, 5766944, 5570083, 5373222, 5176617, 4979756, 4717615, 4520753, 4324148, 4127287, 3930682, 3733821, 3471679, 3274818, 3078213, 2881352, 2684747, 2487886, 2225744, 2028883, 1832278, 1635417, 1438556, 1241950, 979553, 782948, 586087, 389482, 192620, 60784, 59509, 57979, 56704, 55173, 53642, 52367, 50836, 49305, 48030, 46499, 44968, 43694, 42163, 40888, 39357, 37826, 36551, 35020, 33489, 32214, 30684, 29409, 27878, 26347, 25072, 23541, 22010, 20735, 19965, 19195, 18426, 17912, 17142, 16372, 15603, 14833, 14319, 13549, 12780, 12010, 11240, 10726, 9957, 9187, 8417, 7647, 7134, 6364, 5594, 4824, 4055, 3541, 2771, 2001, 1232, 462]  # Seis(256)
          }
          frame "InvertSeis" {
            w117 = u32[] [462, 1232, 2001, 2771, 3541, 4055, 4824, 5594, 6364, 7134, 7647, 8417, 9187, 9957, 10726, 11240, 12010, 12780, 13549, 14319, 14833, 15603, 16372, 17142, 17912, 18426, 19195, 19965, 20735, 22010, 23541, 25072, 26347, 27878, 29409, 30684, 32214, 33489, 35020, 36551, 37826, 39357, 40888, 42163, 43694, 44968, 46499, 48030, 49305, 50836, 52367, 53642, 55173, 56704, 57979, 59509, 60784, 192620, 389482, 586087, 782948, 979553, 1241950, 1438556, 1635417, 1832278, 2028883, 2225744, 2487886, 2684747, 2881352, 3078213, 3274818, 3471679, 3733821, 3930682, 4127287, 4324148, 4520753, 4717615, 4979756, 5176617, 5373222, 5570083, 5766944, 6029086, 6422301, 6749980, 7143195, 7536410, 7929625, 8322840, 8650518, 9043733, 9436948, 9830163, 10223378, 10551057, 10944272, 11337487, 11730702, 12123917, 12451596, 12844811, 13238026, 13631241, 14024456, 14352135, 14745350, 15138565, 15531779, 15924994, 16252673, 16645888, 16776960, 16776960, 16776960, 16776960, 16776960, 16776960, 16776960, 16776960, 16776960, 16776960, 16776960, 16776960, 16776960, 16776960, 16776960, 16776960, 16776960, 16776960, 16776960, 16776960, 16776960, 16776960, 16776960, 16776960, 16776960, 16776960, 16776960, 16776960, 16776704, 16775936, 16775168, 16774400, 16773632, 16772864, 16772096, 16771328, 16770560, 16769792, 16769024, 16768256, 16767488, 16766720, 16765952, 16765184, 16764416, 16763648, 16762880, 16762112, 16761344, 16760576, 16759808, 16759040, 16758272, 16757504, 16756736, 16755968, 16755200, 16754432, 16753664, 16752896, 16752128, 16751360, 16750592, 16749824, 16749056, 16748288, 16747520, 16746752, 16745984, 16745216, 16744448, 16743936, 16743168, 16742400, 16741632, 16740864, 16740096, 16739328, 16738560, 16737792, 16737024, 16736256, 16735488, 16734720, 16733952, 16733184, 16732416, 16731648, 16730880, 16730112, 16729344, 16728576, 16727808, 16727040, 16726272, 16725504, 16724736, 16723968, 16723200, 16722432, 16721664, 16720896, 16720128, 16719360, 16718592, 16717824, 16717056, 16716288, 16715520, 16714752, 16713984, 16713216, 16712448, 16711680, 16515072, 16318464, 16121856, 15925248, 15728640, 15532032, 15335424, 15138816, 14942208, 14745600, 14548992, 14352384, 14155776, 13959168, 13762560, 13565952, 13369344, 13172736, 12976128, 12779520, 12582912, 12386304, 12189696, 11993088, 11796480, 11599872, 11403264, 11206656]  # InvertSeis(256)
          }
          frame "Jaisnd" {
            w118 = u32[] [3014783, 2949253, 2818187, 2621584, 2424982, 2228379, 2031776, 1769637, 1507497, 1245358, 917682, 655542, 327866, 190, 1218, 2757, 4041, 5580, 6863, 8402, 9941, 11480, 12763, 14301, 15840, 17378, 18916, 20198, 21736, 23274, 24556, 25837, 27375, 28656, 29938, 31219, 32500, 33781, 35062, 36343, 37368, 38649, 39673, 40698, 41723, 42747, 43772, 44796, 45821, 46589, 47613, 48381, 49406, 50174, 50942, 51710, 52478, 53502, 54270, 55038, 55806, 122110, 122878, 188926, 189695, 255999, 322303, 388607, 454911, 521215, 587519, 653823, 720127, 851966, 917499, 1048568, 1114101, 1245170, 1376239, 1441772, 1572841, 1703910, 1900515, 2031584, 2162653, 2293722, 2490327, 2621396, 2818001, 3014606, 3145676, 3342281, 3538886, 3735492, 3932097, 4194239, 4390845, 4587451, 4849593, 5046199, 5308341, 5570484, 5832626, 6029233, 6356912, 6619055, 6881199, 7143343, 7471022, 7733166, 8060847, 8388527, 8716208, 9043890, 9371571, 9764789, 10158007, 10485690, 10878908, 11337664, 11730884, 12189640, 12648397, 13172690, 13762520, 14352351, 15073256, 15990772, 16515059, 16318437, 16121818, 15990737, 15925192, 15859648, 15794105, 15794098, 15728556, 15728549, 15728543, 15794074, 15794068, 15859598, 15925129, 15925124, 15990655, 16056186, 16121717, 16252785, 16318316, 16383848, 16514916, 16580448, 16711515, 16776792, 16776276, 16775760, 16775244, 16774985, 16774469, 16773954, 16773439, 16772923, 16772408, 16771893, 16771378, 16770863, 16770093, 16769578, 16769063, 16768549, 16767778, 16767264, 16766750, 16765980, 16765465, 16764695, 16763925, 16763412, 16762642, 16761872, 16761103, 16760333, 16759564, 16758538, 16757769, 16757000, 16755975, 16755206, 16754181, 16753156, 16752131, 16751106, 16684546, 16683521, 16682497, 16681472, 16680192, 16679168, 16677888, 16676608, 16675328, 16674048, 16672768, 16671488, 16604672, 16603136, 16601856, 16600320, 16533248, 16531712, 16464640, 16463104, 16396032, 16328960, 16327168, 16260096, 16192768, 16125696, 16058368, 15991296, 15925252, 15859722, 15728657, 15663128, 15532062, 15466533, 15335467, 15204401, 15073335, 14942269, 14811203, 14680137, 14483535, 14352468, 14155865, 13959262, 13762659, 13566056, 13369452, 13172848, 12910708, 12714103, 12451962, 12189821, 11927679, 11665537, 11403394, 11075716, 10813572, 10485893, 10158212, 9830532, 9437315, 9109633, 8716415, 8323197]  # Jaisnd(256)
          }
          frame "TBD1" {
          }
        }
        n54 = property on="Intensity Graph" class="IntGraph (strict)"("Color Table"=w108) -> ()  [unwired: 2 in, 2 out]
      }
      event "Start": Value Change {
        n55 = event-data() -> ()  [unwired: 1 in, 2 out]
        n56 = property on="Start" class="Bool"("Visible"=FALSE) -> ()  [unwired: 2 in, 2 out]
        n57 = Bundle By Name(cluster=T13 {"State"=enum."Open", "Para."=variant} ("element"), "Para."=w121) -> (w122:T13)
        n58 = Enqueue Element At Opposite End(queue=w125, element=w122) -> (queue out=w123:refnum<queue>)  [unwired: 2 in, 2 out]
      }
    }
  }
  n59 = while {
    shift-right: [w142] -> _
    shift-left: w38 -> [w149]
    shift-right: [w141] -> _
    shift-left: _ -> [w148]
    tunnel: w31 -> [w147]
    tunnel: w44 -> [w145]
    tunnel: "Dynamic Params queue" -> [w138]
    shift-right: [w139] -> _
    shift-left: _ -> [w137]
    shift-right: [w136] -> _
    shift-left: _ -> [w135]
    tunnel: "Quit_UserEvent" -> [w134]
    shift-right: [w132] -> w17
    shift-left: w23 -> [w133]
    shift-right: [w128] -> _
    shift-left: w22 -> [w131]
    shift-right: [w129] -> _
    shift-left: T9 {"File Header"={"Start Position"=[], "StepWidth"=[], "Dimension"=[], "SpecLength"=0}, "mzCali."=[], "m/z_Array"=[], "SampleRate"=100000000.0, "TrigDelay"=0.0, "file refnum"=refnum, "file path"=path "", "PeakOI"=[]} ("output cluster") -> [w130]
    border: w21 -> [_]
    border: ProcessStates."Initialize" -> [_]
    i -> [w126]
    stop <- w140 stop-if-true
    n60 = Dequeue Element(queue=w147) -> (queue out=w143:refnum<queue>, element=w144:T13, error out=w146:errorcluster)  [unwired: 2 in, 1 out]
    n61 = Unbundle By Name(w144) -> ("State"=w127:T26)
    "State" <- w127
    n62 = case shown="No Error" w146 {
      tunnel: w149 -> [w171 w879]
      tunnel: [w170 w879] -> w142
      tunnel: w148 -> [w169 w878]
      tunnel: [w168 w878] -> w141
      tunnel: w145 -> [w167 _]
      tunnel: w127 -> [w166 _]
      tunnel: w144 -> [w165 _]
      tunnel: w143 -> [w164 _]
      tunnel: [w163 TRUE] -> w140
      tunnel: [w162 w876] -> w139
      tunnel: w138 -> [w161 _]
      tunnel: w137 -> [w160 w876]
      tunnel: [w159 w875] -> w136
      tunnel: w135 -> [w158 w875]
      tunnel: w134 -> [w157 _]
      tunnel: w133 -> [w156 w874]
      tunnel: [w150 w874] -> w132
      tunnel: w131 -> [w155 w872]
      tunnel: w130 -> [w154 w873]
      tunnel: [w153 w873] -> w129
      tunnel: [w152 w872] -> w128
      frame No Error {
        n63 = case "Proc. Core" shown="\"Save_Image\"" w166 {
          selector: w166 -> [_ w182 w257 w318 _ w557 w576 _ _ _ _ _]
          tunnel: w171 -> [w178 w192 w236 w332 w372 w556 w581 w597 w619 w670 w694 w744]
          tunnel: [w178 w192 w264 w314 w373 w556 w581 w597 w619 w670 w694 w744] -> w170
          tunnel: [w177 w201 0 w312 w408 w534 w573 w600 w623 w669 w693 w743] -> w168
          tunnel: w169 -> [w177 w201 _ w312 w408 w533 w573 w600 w623 w669 w693 w743]
          tunnel: w167 -> [_ _ _ _ w404 w535 _ _ _ w667 _ _]
          tunnel: w165 -> [_ w183 w225 w320 w406 w558 w577 _ _ _ w685 w735]
          tunnel: w164 -> [_ w184 w258 w321 w407 w559 w578 w596 _ _ _ _]
          tunnel: [_ _ _ _ _ _ _ _ _ TRUE _ _] -> w163
          tunnel: [w176 w200 w235 w316 w405 w548 w575 w595 w617 w666 w688 w738] -> w162
          tunnel: w161 -> [_ _ _ w323 _ _ _ _ _ w659 _ _]
          tunnel: w160 -> [w176 w200 _ w316 w405 w549 w575 w595 w617 w666 w688 w738]
          tunnel: [w175 w199 w253 w313 w387 w555 w574 w594 w609 w665 w692 w742] -> w159
          tunnel: w158 -> [w175 w199 _ w313 w387 w555 w574 w594 w609 w665 w692 w742]
          tunnel: w157 -> [_ _ _ _ _ _ _ _ _ w664 _ _]
          tunnel: w156 -> [w174 w198 w238 w311 w403 _ w572 w592 w608 w654 w691 w741]
          tunnel: [w174 w198 w239 w310 w403 w542 w572 w592 w607 w655 w691 w741] -> w151
          tunnel: w155 -> [w172 w196 w245 w308 w399 w551 w570 w590 _ w657 w689 w739]
          tunnel: w154 -> [w173 w197 w223 w309 w374 w545 w571 w591 w606 w658 w690 w740]
          tunnel: [w173 w194 w242 w309 w374 w547 w571 w591 _ w658 w690 w740] -> w153
          tunnel: [w172 w195 w245 w308 w400 w551 w570 w590 _ w657 w689 w739] -> w152
          frame Default {
          }
          frame "Initialize" {
            w185 = cluster{"m/z":dbl, "Width(+/-)":dbl}[] [{"m/z"=110.0, "Width(+/-)"=100.0}]  # 10-210 as default range
            w193 = u32[] [0, 0, 12517567, 12320960, 12189888, 12058817, 11927746, 11731139, 11600067, 9175197, 9044125, 11141318, 11010246, 10813639, 10682568, 10551497, 10354890, 10223818, 10092747, 7930019, 7798948, 9633997, 9502926, 9306319, 9175248, 9044176, 8847569, 8716498, 8585427, 6750377, 6619306, 8126677, 7995606, 7798999, 7667927, 7536856, 7340249, 7209178, 7078106, 5505199, 5374128, 6619357, 6488285, 6291678, 6160607, 6029536, 5832929, 5701857, 5570786, 4325557, 4194486, 5112036, 4980965, 4784358, 4653287, 4522215, 4325608, 4194537, 4063466, 3080380, 3014844, 3604716, 3408109, 3277038, 3277038, 3145966, 3014895, 2818288, 2687217, 2556145, 1900738, 1769666, 2097396, 1900789, 1769717, 1638646, 1507575, 1310968, 1179896, 1048825, 721096, 590024, 590075, 393468, 262397, 131326, 255, 1791, 3327, 4863, 5068, 6348, 9471, 11007, 12543, 14079, 15615, 17151, 18687, 20223, 17612, 18636, 25087, 26623, 28159, 29695, 31231, 32767, 34303, 35839, 29900, 31180, 40447, 41983, 43775, 45311, 46847, 48383, 49919, 51455, 42444, 43724, 56063, 57599, 59135, 60671, 62207, 63743, 65535, 65528, 52418, 52413, 65510, 65504, 65498, 65492, 65486, 65480, 65474, 65468, 52369, 52364, 65449, 65443, 65437, 65431, 65425, 65419, 65413, 65407, 52321, 52316, 65389, 65383, 65377, 65371, 65364, 65358, 65352, 65346, 52272, 52267, 65328, 65322, 65316, 65310, 65304, 65298, 65292, 65286, 52224, 314368, 851712, 1244928, 1638144, 2031360, 2424576, 2817792, 3211008, 3604224, 3197952, 3525632, 4783872, 5177088, 5635840, 6029056, 6422272, 6815488, 7208704, 7601920, 6409216, 6736896, 6736896, 8781568, 9174784, 9568000, 9961216, 10354432, 10747648, 11206400, 11599616, 9554944, 9882624, 12779264, 13172480, 13565696, 13958912, 14352128, 14745344, 15138560, 15531776, 12766208, 13093888, 16776960, 16775170, 16773637, 16771847, 16770314, 16768780, 16766991, 16765457, 13411088, 13409810, 16760601, 16758812, 16757278, 16755745, 16753955, 16752422, 16750888, 16749099, 13398052, 13396774, 16744243, 16742704, 16741166, 16739884, 16738345, 16736807, 16735269, 16733730, 13385753, 13384728, 16729371, 16727833, 16726295, 16725012, 16723474, 16721936, 16720397, 16718859, 13373959, 13372677, 16714500, 16712962, 16777215]  # Color table (Rainbow-striped)
            n64 = disable-structure "Wait for manual start signal" shown="Enabled" {
              disable-tunnel: w184 -> [w204 _]
              disable-tunnel: w183 -> [w203 _]
              disable-tunnel: w182 -> [w202 _]
              frame Disabled {
                n65 = Increment(x=w202) -> (x+1=w205:T26)
                n66 = Bundle By Name(cluster=w203, "State"=w205) -> (w206:T13)
                n67 = Enqueue Element(queue=w204, element=w206) -> ()  [unwired: 2 in, 3 out]
              }
              frame Enabled {
              }
            }
            n68 = Unbundle By Name(w192) -> ("File Header.SpecLength"=w187:i32, "File Header"=w181:T10, "mzCali."=w190:dbl[], "SampleRate"=w188:T11, "TrigDelay"=w189:dbl)
            n69 = Subtract(x=w187, y=64) -> (x-y=w179:i32)
            n70 = in-place "Compensate error in float-point number calculation" {
              n71 = in-place-cluster #1(w181) -> ("StepWidth"=w207:dbl[], "Start Position"=w212:dbl[])
              n72 = Index Array(array=w207) -> (element=w211:dbl)  [unwired: 1 in]
              n73 = Multiply(x=w211, y=0.001) -> (x*y=w209:dbl)
              n74 = in-place {
                in-place-border: w209 -> [w214]
                n75 = in-place-array #2(w212, 0) -> (w215:dbl)
                n76 = Subtract(x=w215, y=w214) -> (x-y=w216:dbl)
                n77 = in-place-array #2(w216) -> (w213:dbl[])  [unwired: 1 out]
              }
              n78 = in-place-cluster #1("StepWidth"=w207, "Start Position"=w213) -> (w180:T10)
            }
            n79 = call "CalcMzArray.vi"("TrigDelay"=w189, "Sample Rate"=w188, "Depth"=w179, "mzCali. (a/b/c)"=w190) -> ("mzArray"=w191:dbl[])  [unwired: 7 in]
            n80 = Bundle By Name(cluster=w197, "File Header.SpecLength"=w179, "m/z_Array"=w191, "File Header"=w180, "mzCali."=w190, "SampleRate"=w188, "TrigDelay"=w189, "PeakOI"=w185) -> (w194:T9)
            n81 = Bundle By Name(cluster=w196, "Depth"=w179) -> (w195:T8)
            n82 = property on="Intensity Graph" class="IntGraph (strict)"("Color Table"=w193) -> ()  [unwired: 2 in, 2 out]
          }
          frame "Open" {
            (unwired) T16 {"queue out"=refnum, "queue out"=refnum} ("output cluster")
            w230 = "ActionCallBack" ("name (unnamed)")
            (unwired) cluster{dbl[], dbl[]}[][] []
            # "8192x32KB*4 = 1GB\n!! attention:\nshould be big"
            n83 = Increment(x=w257) -> (x+1=w259:T26)
            n84 = Unbundle By Name(w223) -> ("PeakOI"=w219:cluster{"m/z":dbl, "Width(+/-)":dbl}[])
            n85 = Unbundle By Name(w225) -> ("Para."=w224:variant)
            n86 = Bundle By Name(cluster=w225, "State"=w259) -> (w260:T13)
            n87 = Variant To Data(type=w219, Variant=w224) -> (data=w221:cluster{"m/z":dbl, "Width(+/-)":dbl}[], error out=w222:errorcluster)  [unwired: 1 in]
            n88 = Enqueue Element(queue=w258, element=w260) -> ()  [unwired: 2 in, 3 out]
            n89 = Select(t=w219, s=w222, f=w221) -> (s? t:f=w220:cluster{"m/z":dbl, "Width(+/-)":dbl}[])
            n90 = while {
              tunnel: [w273] -> w241
              tunnel: [w272] -> w243
              tunnel: [w271] -> w240
              tunnel: [w270] -> w239
              tunnel: w238 -> [w269]
              stop <- w274 stop-if-true
              n91 = Not A Number/Path/Refnum?(number/path/refnum="BioMAP file path") -> (NaN/Path/Refnum?=w266:bool)
              n92 = feedback #3(path "" ("selected path")) -> (w278:path)
              n93 = case shown="False" w266 {
                tunnel: w278 -> [_ w290]
                tunnel: [w281 w289] -> w276
                tunnel: [FALSE ("cancelled") w288] -> w275
                tunnel: w269 -> [w279 w287]
                tunnel: [w279 w286] -> w268
                tunnel: "BioMAP file path" -> [w281 _]
                frame False {
                }
                frame True {
                  n94 = Strip Path(path=w290) -> (stripped path=w283:path, name=w284:string)
                  n95 = call "File Dialog2"("start path"=w283, "default name"=w284, "error in"=w287, "pattern (all files)"="*.img", "pattern label"="BioMAP Analyze v7.5") -> ("selected path"=w289:path, "cancelled"=w288:bool, "error out"=w286:errorcluster)  [unwired: 7 in, 1 out]
                }
              }
              n96 = case shown="False" w275 {
                tunnel: w276 -> [w298 _]
                tunnel: [w298 w305] -> w277
                tunnel: w278 -> [_ w305]
                tunnel: [w293 w304] -> w274
                tunnel: [w298 path "" ("selected path")] -> w273
                tunnel: [w293 _] -> w272
                tunnel: [w295 _] -> w271
                tunnel: [w292 errorcluster {"status"=FALSE, "code"=0, "source"=""} ("error out")] -> w270
                tunnel: w268 -> [w291 _]
                frame False {
                  n97 = Open/Create/Replace File(file path (use dialog)=w298, error in=w291, operation (0:open)=T20."replace or create", access (0:read/write)=enum16{"read/write", "read-only", "write-only"}."write-only") -> (refnum out=w295:refnum<file>, cancelled=w294:bool, error out=w292:errorcluster)  [unwired: 2 in]
                  n98 = Compound Arithmetic op=AND(invert w294, TRUE) -> (w293:bool)
                  "Export File Path" <- w298
                }
                frame True {
                  n99 = Two Button Dialog(message="Continue without saving?", 1:"No saving" ("F button name (\"Cancel\")"), 2:"Set Filename" ("T button name (\"OK\")")) -> (T button?=w306:bool)
                  n100 = Not(x=w306) -> (.not. x?=w304:bool)
                }
              }
              n101 = feedback-in #3(w277) -> ()
            }
            n102 = Obtain Queue(max queue size (-1, unlimited)=32768, name (unnamed)="BeamProfiling_Buffer", element data type=T18 {"SampleRate"=0.0, "TrigDelay"=0.0, "SpecLength"=0.0, "DAQ_Range"=0.0, "Average#"=0, "Position"=[], "Spectrum"=[], "Calibr."=[], "Pressure"=0.0, "Desp_LaserEnergy"=0.0, "PI_LaserEnergy"=0.0, "Voltages Table"=[], "ProcMode"=enum."None", "Threshold"=0.0, "Comment"="", "TickCount"=0.0, "Time Stamp"=timestamp(0 s since 1904-01-01)} ("Signal Segment")) -> (queue out=w253:refnum<queue>, error out=w252:errorcluster)  [unwired: 2 in, 1 out]
            n103 = Obtain Queue(name (unnamed)=w230, element data type=w230) -> (queue out=w227:refnum<queue>)  [unwired: 3 in, 2 out]
            n104 = Bundle(cluster=T16 {"queue out"=refnum, "queue out"=refnum}, "queue out"=w253, "queue out"=w227) -> (w237:T16)
            n105 = Unbundle By Name(w236) -> ("ControlRefs.ProcCore_CtrlQueue"=w254:refnum<queue>)
            n106 = Bundle By Name(cluster=T17 {"Command"=enum."SetWriterRef", "Params"=variant} ("element"), "Command"=ProcessStates."SetWriterRef", "Params"=w237) -> (w262:T17)
            n107 = Unbundle By Name(w223) -> ("File Header.Dimension"=w233:i32[])
            n108 = Enqueue Element "Set Data queue"(queue=w254, element=w262, error in (no error)=w252) -> (queue out=w247:refnum<queue>, error out=w229:errorcluster)  [unwired: 1 in, 1 out]
            n109 = Index Array(array=w233) -> (element #1=w232:i32, element #2=w231:i32)  [unwired: 2 in]
            n110 = Dequeue Element(queue=w227, error in (no error)=w229) -> (error out=w228:errorcluster)  [unwired: 1 in, 3 out]
            n111 = Bundle By Name(cluster=T17 {"Command"=enum."SetWriterRef", "Params"=variant} ("element"), "Command"=ProcessStates."StartSave") -> (w249:T17)
            n112 = Initialize Array(0.0, w232, w231, 10 ("dimension size")) -> (w235:dbl[][][])
            n113 = Enqueue Element "Start Send Data"(queue=w247, element=w249, error in (no error)=w228) -> (error out=w246:errorcluster)  [unwired: 1 in, 2 out]
            n114 = call <vilib>:"Clear Errors.vi"("error in (no error)"=w246) -> ()  [unwired: 6 in, 1 out]
            n115 = Bundle By Name(cluster=w223, "PeakOI"=w220, "file path"=w241, "file refnum"=w240) -> (w242:T9)
            n116 = Bundle By Name(cluster=w236, "Scan#"=0, "Save?"=w243) -> (w264:T14)
          }
          frame "PrepScanParams" {
            n117 = Increment(x=w318) -> (x+1=w317:T26)
            n118 = Bundle By Name(cluster=w320, "State"=w317) -> (w319:T13)
            n119 = Unbundle By Name(w332) -> ("Scan#"=w324:i32)
            n120 = Enqueue Element(queue=w321, element=w319) -> ()  [unwired: 2 in, 3 out]
            n121 = Equal To 0?(x=w324) -> (x = 0?=w333:bool)
            n122 = Increment(x=w324) -> (x+1=w331:i32)
            n123 = case shown="True" w333 {
              tunnel: w332 -> [w345 w369]
              tunnel: [w335 w364] -> w329
              tunnel: [w339 w368] -> w328
              tunnel: [w338 w367] -> w327
              tunnel: [w337 w366] -> w326
              tunnel: w324 -> [_ w365]
              tunnel: w312 -> [_ _]
              frame True {
                w334 = 0
                # "Initial scan, stick to orignal parameter"
                n124 = Unbundle By Name(w345) -> ("HighSpeed"=w338:dbl, "ScanSpeed"=w337:dbl, "File Header"=w340:T10)
                n125 = Unbundle By Name(w340) -> ("Start Position"=w335:dbl[], "StepWidth"=w343:dbl[], "Dimension"=w344:i32[])
                n126 = Index Array(array=w343, index=w334) -> (element=w342:dbl)
                n127 = Index Array(array=w344, index=w334) -> (element=w341:i32)
                n128 = Multiply(x=w342, y=w341) -> (x*y=w336:dbl)
                n129 = in-place {
                  in-place-border: w336 -> [w347]
                  n130 = in-place-array #4(w335, w334) -> (w348:dbl)
                  n131 = Add(x=w348, y=w347) -> (x+y=w346:dbl)
                  n132 = in-place-array #4(w346) -> (w339:dbl[])  [unwired: 1 out]
                }
              }
              frame False {
                w349 = 1
                w355 = 0 ("index")
                n133 = Unbundle By Name(w369) -> ("HighSpeed"=w367:dbl, "ScanSpeed"=w366:dbl, "File Header"=w357:T10)
                n134 = Unbundle By Name(w357) -> ("Start Position"=w350:dbl[], "StepWidth"=w362:dbl[], "Dimension"=w363:i32[])
                n135 = Index Array(array=w350, index #1=w355, index #2=w349) -> (element #1=w361:dbl, element #2=w352:dbl)
                n136 = Index Array(array=w362, index #1=w355, index #2=w349) -> (element #1=w359:dbl, element #2=w354:dbl)
                n137 = Index Array(array=w363, index=w355) -> (element=w358:i32)
                n138 = Multiply(x=w359, y=w358) -> (x*y=w360:dbl)
                n139 = Multiply(x=w354, y=w365) -> (x*y=w353:dbl)
                n140 = Add(x=w361, y=w360) -> (x+y=w356:dbl)
                n141 = Add(x=w352, y=w353) -> (x+y=w351:dbl)
                n142 = in-place {
                  in-place-border: w356 -> [w371]
                  in-place-border: w351 -> [w370]
                  n143 = in-place-array #5(w350, w349) -> ()  [unwired: 1 out]
                  n144 = in-place-array #6(w350, w355, w349) -> ()  [unwired: 2 out]
                  n145 = in-place-array #5(w370) -> (w364:dbl[])  [unwired: 1 out]
                  n146 = in-place-array #6(w371, w370) -> (w368:dbl[])  [unwired: 2 out]
                }
              }
            }
            n147 = Bundle By Name(cluster=w332, "Scan#"=w331) -> (w314:T14)
            n148 = Bundle By Name(cluster=T21 {"Start Position"=[], "End Position"=[], "HighSpeed"=0.0, "ScanSpeed"=0.0, "KeepStill(ms)"=0}, "HighSpeed"=w327, "ScanSpeed"=w326, "Start Position"=w329, "End Position"=w328, "KeepStill(ms)"=u32 0 ("Wait(ms)")) -> (w322:T21)
            n149 = Enqueue Element "Send scan params"(queue=w323, element=w322) -> (error out=w315:errorcluster)  [unwired: 2 in, 2 out]
            n150 = Merge Errors(w315, w311) -> (w310:errorcluster)
            n151 = call <vilib>:"Clear Errors.vi"("error in (no error)"=w315) -> ()  [unwired: 6 in, 1 out]
          }
          frame "WaitData" {
            # "Need EOF detection, \nAnd set Y Dimension to current value"
            # "Need detection of EOF"
            # "TODO:  Remove average forcing 1 to sum true average#!!"
            n152 = Dequeue Element "WaitSpectra"(queue=w387) -> (element=w401:T18)  [unwired: 2 in, 3 out]
            n153 = Unbundle By Name(w401) -> ("TickCount"=w381:dbl, "Position"=w392:dbl[], "Spectrum"=w385:sgl[], "Average#"=w383:i32, "Comment"=w378:string)
            n154 = Search and Replace String(input string=w378, search string="EOF" ("y")) -> (number of replacements=w376:i32)  [unwired: 6 in, 3 out]
            n155 = String Subset(string=w378, length (rest)=2 ("length (rest)")) -> (substring=w382:string)  [unwired: 1 in]
            n156 = Type Cast(type=ProcessStates."StartOfLine", x=w382) -> (*(type *) &x=w389:T7)
            n157 = Unbundle By Name(w374) -> ("File Header.Start Position"=w390:dbl[], "File Header.StepWidth"=w391:dbl[])
            n158 = Greater Than 0?(x=w376) -> (x > 0?=w375:bool)
            n159 = Select(t=ProcessStates."Quit", s=w375, f=w389) -> (s? t:f=w380:T7)
            n160 = feedback-in #7(w380) -> ()
            n161 = feedback #7() -> (w388:T7)
            n162 = Multiply(x=w385, y=w383) -> (x*y=w384:sgl[])
            n163 = case "Average Spectra in a single pixel" shown="Default" w380 {
              tunnel: w407 -> [w432 w454 w466 w497]
              tunnel: w404 -> [w429 w451 w464 w494]
              tunnel: w406 -> [_ _ w465 w496]
              tunnel: w399 -> [w428 w450 _ w495]
              tunnel: [_ _ _ w493] -> w400
              tunnel: [w427 w449 _ w492] -> w393
              tunnel: w384 -> [_ _ _ w479]
              tunnel: w392 -> [_ _ _ w478]
              tunnel: w391 -> [_ _ _ w477]
              tunnel: w390 -> [_ _ _ w476]
              tunnel: w388 -> [_ _ _ w473]
              tunnel: [_ _ _ w471] -> _
              tunnel: w383 -> [_ _ _ w468]
              tunnel: w381 -> [_ _ _ _]
              tunnel: [w415 w443 w460 w467] -> w373
              tunnel: w372 -> [w415 w442 w460 w467]
              frame "EndOfLine" {
                # "Dealing with ocassional corrupted data"
                # "End of Line"
                n164 = Unbundle By Name(w428) -> ("Average"=w430:i32, "Spectra"=w431:sgl[])  [unwired: 1 out]
                n165 = Get Queue Status(queue=w429) -> (queue out=w423:refnum<queue>, # elements in queue=w422:i32)  [unwired: 2 in, 6 out]
                n166 = To Single Precision Float(number=w431) -> (single precision float=w426:sgl[])
                n167 = To Single Precision Float(number=w430) -> (single precision float=w425:sgl)
                n168 = Less?(x=w422, y=5) -> ()  [unwired: 1 out]
                n169 = Divide(x=w426, y=w425) -> (x/y=w427:sgl[])
                n170 = Bundle By Name(cluster=w428, "Average"=w430, "Spectra"=w427) -> (w424:T8)
                n171 = case shown="False" FALSE {
                  tunnel: w424 -> [w435 _]
                  tunnel: w423 -> [w434 w437]
                  tunnel: [T13 {"State"=enum."Flush", "Para."=variant} ("element") T13 {"State"=enum."WaitData", "Para."=variant} ("element")] -> w420
                  frame False {
                    n172 = Enqueue Element(queue=w434, element=w435) -> ()  [unwired: 2 in, 3 out]
                  }
                  frame True {
                    n173 = Flush Queue(queue=w437) -> ()  [unwired: 1 in, 3 out]
                  }
                }
                n174 = Enqueue Element At Opposite End(queue=w432, element=w420) -> ()  [unwired: 2 in, 3 out]
                n175 = feedback #8(0) -> (w418:i32)
                n176 = Increment(x=w418) -> (x+1=w417:i32)
                "#EOL" <- w417
                n177 = feedback-in #8(w417) -> ()
              }
              frame "Quit" {
                # "For incomplete files"
                # "End of File detected"
                n178 = Unbundle By Name(w450) -> ("Average"=w452:i32, "Spectra"=w453:sgl[])  [unwired: 1 out]
                n179 = disable-structure shown="Enabled" {
                  disable-tunnel: w454 -> [w458 w459]
                  disable-tunnel: [w457 w459] -> w444
                  frame Disabled {
                    n180 = Enqueue Element At Opposite End(queue=w458, element=T13 {"State"=enum."Close", "Para."=variant}) -> (queue out=w457:refnum<queue>)  [unwired: 2 in, 2 out]
                  }
                  frame Enabled {
                  }
                }
                n181 = To Single Precision Float(number=w453) -> (single precision float=w448:sgl[])
                n182 = To Single Precision Float(number=w452) -> (single precision float=w447:sgl)
                n183 = Unbundle By Name(w442) -> ("File Header.Dimension"=w441:i32[], "Scan#"=w438:i32)
                n184 = Divide(x=w448, y=w447) -> (x/y=w449:sgl[])
                n185 = Bundle By Name(cluster=w450, "Average"=w452, "Spectra"=w449) -> (w446:T8)
                n186 = Enqueue Element(queue=w451, element=w446) -> ()  [unwired: 2 in, 3 out]
                n187 = in-place {
                  in-place-border: w438 -> [w455]
                  n188 = in-place-array #9(w441, 1) -> ()  [unwired: 1 out]
                  n189 = in-place-array #9(w455) -> (w440:i32[])  [unwired: 1 out]
                }
                n190 = Enqueue Element At Opposite End(queue=w444, element=T13 {"State"=enum."Flush", "Para."=variant}) -> ()  [unwired: 2 in, 3 out]
                n191 = Bundle By Name(cluster=w442, "File Header.Dimension"=w440) -> (w443:T14)
              }
              frame "StartOfLine" {
                # "New Line"
                n192 = Enqueue Element "Implied \"WaitData\""(queue=w466, element=w465) -> ()  [unwired: 2 in, 3 out]
                n193 = Flush Queue(queue=w464) -> ()  [unwired: 1 in, 3 out]
                n194 = feedback #10(0) -> (w462:i32)
                n195 = Increment(x=w462) -> (x+1=w461:i32)
                "#SOL" <- w461
                n196 = feedback-in #10(w461) -> ()
              }
              frame Default {
                # "Normal Spectra"
                n197 = Index Array(array=w476) -> (element #1=w487:dbl, element #2=w488:dbl)  [unwired: 2 in]
                n198 = Index Array(array=w477) -> (element #1=w489:dbl, element #2=w490:dbl)  [unwired: 2 in]
                n199 = Index Array(array=w478) -> (element #1=w472:dbl, element #2=w491:dbl)  [unwired: 2 in]
                n200 = Enqueue Element "Implied \"WaitData\""(queue=w497, element=w496) -> ()  [unwired: 2 in, 3 out]
                n201 = Subtract "Y"(x=w491, y=w488) -> (x-y=w484:dbl)
                n202 = Subtract "X"(x=w472, y=w487) -> (x-y=w485:dbl)
                n203 = Divide(x=w484, y=w490) -> (x/y=w483:dbl)
                n204 = Divide(x=w485, y=w489) -> (x/y=w486:dbl)
                n205 = Round Toward -Infinity(1:w486) -> (0:w481:dbl)
                n206 = Round Toward -Infinity(1:w483) -> (0:w482:dbl)
                n207 = To Long Integer(number=w481) -> (32bit integer=w469:i32)
                n208 = To Long Integer(number=w482) -> (32bit integer=w470:i32)
                n209 = call-poly <userlib>:"Data Changed__ogtk.vi"("I32"=w470) -> ("Changed"=w471:bool)
                n210 = Bundle By Name(cluster=T8 {"Average"=0, "X (Img)"=0, "Y (Img)"=0, "Spectra"=[], "Depth"=0} ("output cluster"), "X (Img)"=w469, "Y (Img)"=w470, "Spectra"=w479, "Average"=w468) -> (w480:T8)
                n211 = call-poly <userlib>:"Data Changed__ogtk.vi"("I32"=w469) -> ("Changed"=w474:bool)
                n212 = case shown="True" w474 {
                  tunnel: w494 -> [_ w518]
                  tunnel: w495 -> [w502 w514]
                  tunnel: [w503 w516] -> w493
                  tunnel: w480 -> [w501 w516]
                  tunnel: [w500 w513] -> w492
                  tunnel: w473 -> [_ w511]
                  frame False {
                    # "To be averaged"
                    n213 = Unbundle By Name(w501) -> ("Spectra"=w498:sgl[], "Average"=w499:i32)
                    n214 = in-place {
                      in-place-border: w498 -> [w509]
                      in-place-border: w499 -> [w507]
                      in-place-border: [w506] -> w500
                      n215 = in-place-cluster #11(w502) -> ("Spectra"=w505:sgl[], "Average"=w504:i32)
                      n216 = Compound Arithmetic op=ADD(w505, w509) -> (w506:sgl[])
                      n217 = Compound Arithmetic op=ADD(w504, w507) -> (w508:i32)
                      n218 = in-place-cluster #11("Spectra"=w506, "Average"=w508) -> (w503:T8)
                    }
                  }
                  frame True {
                    # "First one of a pixel"
                    n219 = Unbundle By Name(w514) -> ("Average"=w515:i32, "Spectra"=w519:sgl[])
                    "# average" <- w515
                    n220 = Not Equal?(x=ProcessStates."StartOfLine", y=w511) -> (x != y?=w510:bool)
                    n221 = To Single Precision Float(number=w519) -> (single precision float=w521:sgl[])
                    n222 = To Single Precision Float(number=w515) -> (single precision float=w520:sgl)
                    n223 = Divide(x=w521, y=w520) -> (x/y=w513:sgl[])
                    n224 = Bundle By Name(cluster=w514, "Average"=w515, "Spectra"=w513) -> (w517:T8)
                    n225 = case shown="True" w510 {
                      tunnel: w518 -> [_ w523]
                      tunnel: w517 -> [_ w522]
                      frame False {
                      }
                      frame True {
                        n226 = Enqueue Element ("Push previous to stack")(queue=w523, element=w522) -> ()  [unwired: 2 in, 3 out]
                      }
                    }
                  }
                }
              }
            }
            n227 = Tick Count (ms)() -> (millisecond timer value=w395:u32)
            n228 = Less?(x=u32 50, y=w395) -> (x < y?=w396:bool)
            n229 = feedback #12() -> (w397:u32)
            n230 = case "raw MS refresh" shown="True" w396 {
              tunnel: w393 -> [_ w413]
              tunnel: w395 -> [_ w414]
              tunnel: [w409 w414] -> w398
              tunnel: w397 -> [w409 _]
              tunnel: w374 -> [_ w411]
              frame False {
              }
              frame True {
                n231 = Unbundle By Name(w411) -> ("m/z_Array"=w412:dbl[])
                n232 = Bundle("m/z_Array"=w412, w413) -> (→"MS (Raw)":cluster{"m/z_Array":dbl[], sgl[]})  [unwired: 1 in]
              }
            }
            n233 = feedback-in #12(w398) -> ()
          }
          frame "Flush" {
            n234 = Preview Queue Element(queue=w559, timeout in ms (-1)=0) -> (queue out=w532:refnum<queue>, element=w529:T13, timed out?=w524:bool, error out=w531:errorcluster)  [unwired: 1 in]
            n235 = Not Equal?(x=T13 {"State"=enum."Close", "Para."=variant}, y=w529) -> (x != y?=w528:cluster{"State":bool, "Para.":bool})
            n236 = Unbundle By Name(w528) -> ("State"=w527:bool)
            n237 = Or(x=w527, y=w524) -> (x .or. y?=w525:bool)
            n238 = case shown="True" w525 {
              tunnel: w558 -> [_ w567]
              tunnel: w557 -> [_ w566]
              tunnel: [w561 w565] -> w541
              tunnel: [w560 w564] -> w539
              tunnel: w532 -> [w561 w563]
              tunnel: w531 -> [w560 w562]
              frame False {
              }
              frame True {
                n239 = Increment(x=w566) -> (x+1=w568:T26)
                n240 = Bundle By Name(cluster=w567, "State"=w568) -> (w569:T13)
                n241 = Enqueue Element(queue=w563, element=w569, error in (no error)=w562) -> (queue out=w565:refnum<queue>, error out=w564:errorcluster)  [unwired: 1 in, 1 out]
              }
            }
            n242 = property on="PeakOI #" class="DigNum (strict)"() -> ("Value"=w536:i32)  [unwired: 2 in, 2 out]
            n243 = Bundle By Name(cluster=T13 {"State"=enum."Refresh_Image", "Para."=variant} ("element"), "Para."=w536) -> (w537:T13)
            n244 = Enqueue Element(queue=w541, element=w537, error in (no error)=w539) -> (error out=w540:errorcluster)  [unwired: 1 in, 2 out]
            n245 = control-ref of="This VI"() -> (w554:refnum<vi>)
            n246 = property class="VI"(reference=w554, error in=w540, "FP:RunTransparently"=FALSE ("Front Panel Window:Run VI Transparently"), "FP:Transparency"=u8 0 ("Front Panel Window:Transparency")) -> (error out=w544:errorcluster)  [unwired: 1 out]
            n247 = Increment(x=w533) -> (x+1=w534:i32)
            n248 = call "BioMapWriteCore.vi"("conv. coeff."="conv. coeff.", "Image in"=w549, "error in"=w544, "Y_img"=w533, "Image Params"=w545, "stack queue in"=w535) -> ("error out"=w543:errorcluster, "file refnum out"=w546:refnum<file>, "Image out"=w548:dbl[][][])  [unwired: 3 in]
            n249 = Bundle By Name(cluster=w545, "file refnum"=w546) -> (w547:T9)
            n250 = call <vilib>:"General Error Handler.vi"("error in (no error)"=w543) -> ("error out"=w542:errorcluster)  [unwired: 10 in, 4 out]
            "Line#" <- w533
          }
          frame "ScanResult" {
            n251 = Increment(x=w576) -> (x+1=w579:T26)
            n252 = Bundle By Name(cluster=w577, "State"=w579) -> (w580:T13)
            n253 = Enqueue Element(queue=w578, element=w580) -> ()  [unwired: 2 in, 3 out]
          }
          frame "CheckEndCondition" {
            w598 = 1  # axis Y
            # "Add condition:\nreader quit due to file ends"
            n254 = Unbundle By Name(w597) -> ("Scan#"=w589:i32, "File Header.Dimension"=w599:i32[])
            n255 = Index Array(array=w599, index=w598) -> (element=w588:i32)
            n256 = Subtract(x=w589, y=w588) -> (x-y=w587:i32)
            n257 = Greater Or Equal?(x=w587, y=0) -> (x >= y?=w593:bool)
            n258 = Negate(x=w587) -> (-x=→"remaining lines":i32)
            n259 = Select(t=T13 {"State"=enum."Close", "Para."=variant}, s=w593, f=T13 {"State"=enum."PrepScanParams", "Para."=variant}) -> (s? t:f=w582:T13)
            n260 = Enqueue Element(queue=w596, element=w582) -> ()  [unwired: 2 in, 3 out]
          }
          frame "Close" {
            n261 = Unbundle By Name(w606) -> ("file path"=w603:path)
            n262 = property on="Cancel" class="Bool"("Visible"=FALSE) -> ()  [unwired: 2 in, 2 out]
            n263 = property on="Close/Quit" class="Bool (strict)"("BoolText.Text"="Done" ("Boolean Text.Text")) -> ()  [unwired: 2 in, 2 out]
            n264 = Not Equal?(x=w603, y=path "" ("file path")) -> (x != y?=w605:bool)
            n265 = case shown="True" w605 {
              tunnel: w608 -> [w624 w637]
              tunnel: w606 -> [_ w631]
              tunnel: [w624 w630] -> w607
              frame False {
              }
              frame True {
                n266 = Unbundle By Name(w631) -> ("file path"=w634:path, "File Header.SpecLength"=w635:i32, "File Header.Dimension"=w636:i32[], "file refnum"=w644:refnum<file>, "m/z_Array"=w627:dbl[], "TrigDelay"=w625:dbl, "SampleRate"=w633:T11, "mzCali."=w626:dbl[])
                "mzCali." <- w626
                n267 = Reciprocal(x=w633) -> (1/x=w632:T11)
                n268 = Close File(refnum=w644, error in=w637) -> (error out=w628:errorcluster)  [unwired: 1 out]
                n269 = disable-structure shown="Enabled" {
                  disable-tunnel: w626 -> [w649 _]
                  disable-tunnel: w635 -> [w648 w650]
                  disable-tunnel: w634 -> [w647 w652]
                  disable-tunnel: w632 -> [w646 _]
                  disable-tunnel: w625 -> [w645 _]
                  disable-tunnel: [_ w653] -> w629
                  disable-tunnel: w627 -> [_ w651]
                  frame Enabled {
                    n270 = call "BioMapT2mWriter.vi"("TrigDelay"=w645, "time bin (s)"=w646, "SpecDepth"=w648, "Cali. Values"=w649, "image file path"=w647) -> ()  [unwired: 6 in, 1 out]
                  }
                  frame Disabled {
                    n271 = call "BioMapT2mWriter(Mapping).vi"("SpecLength"=w650, "mzArray"=w651, "image file path"=w652) -> ("error out"=w653:errorcluster)  [unwired: 8 in]
                  }
                }
                n272 = Index Array(array=w636) -> (element #1=w639:i32, element #2=w638:i32)  [unwired: 2 in]
                n273 = Bundle By Name(cluster=T22 {"Dimension"=4, "SpecDepth"=0, "x dimension"=0, "y dimension"=0, "z dimension"=1} ("Dimensions"), "SpecDepth"=w635, "x dimension"=w639, "y dimension"=w638) -> (w643:T22)
                n274 = call "BioMapHeaderWriter.vi"("Pixel Dimension"=T23 {"Dimension 1"=1.0, "Dimension 2"=1.0, "Dimension 3"=1.0, "Dimension 4"=1.0, "Dimension 5"=0.0, "Dimension 6"=0.0, "Dimension 7"=0.0, "Dimension 8"=0.0}, "Dimensions"=w643, "image file path"=w634) -> ("error out"=w640:errorcluster)  [unwired: 8 in]
                n275 = Merge Errors(w640, w629, w628) -> (w630:errorcluster)
              }
            }
            n276 = Unbundle By Name(w619) -> ("ControlRefs.ProcCore_CtrlQueue"=w614:refnum<queue>, "ControlRefs.WriterSIG"=w618:refnum<queue>)
            n277 = Bundle By Name(cluster=T17 {"Command"=enum."SetWriterRef", "Params"=variant} ("element"), "Command"=ProcessStates."StopSave") -> (w613:T17)
            n278 = Bundle By Name(cluster=T17 {"Command"=enum."SetWriterRef", "Params"=variant} ("element"), "Command"=ProcessStates."SetWriterRef", "Params"=w618) -> (w621:T17)
            n279 = Enqueue Element(queue=w614, element=w613) -> (queue out=w612:refnum<queue>, error out=w611:errorcluster)  [unwired: 2 in, 1 out]
            n280 = Enqueue Element(queue=w612, element=w621, error in (no error)=w611) -> (error out=w610:errorcluster)  [unwired: 1 in, 2 out]
            n281 = call <vilib>:"Clear Errors.vi"("error in (no error)"=w610) -> ()  [unwired: 6 in, 1 out]
          }
          frame "Quit" {
            n282 = disable-structure shown="Enabled" {
              disable-tunnel: w659 -> [w673 _]
              frame Enabled {
                # "Bad solution: have upper level jump out wait queue"
                n283 = Enqueue Element(queue=w673, element=T21 {"Start Position"=[], "End Position"=[], "HighSpeed"=0.0, "ScanSpeed"=0.0, "KeepStill(ms)"=0}) -> (error out=w671:errorcluster)  [unwired: 2 in, 2 out]
                n284 = call <vilib>:"Clear Errors.vi"("error in (no error)"=w671) -> ()  [unwired: 6 in, 1 out]
              }
              frame Disabled {
              }
            }
            n285 = Release Queue(queue=w667, error in (no error)=w654) -> (error out=w656:errorcluster)  [unwired: 1 in, 2 out]
            n286 = Generate User Event(user event=w664, event data cluster=cluster{bool} {TRUE} ("event data")) -> (user event out=w662:refnum<user-event>, error out=w661:errorcluster)  [unwired: 2 in]
            n287 = Destroy User Event(user event=w662, error in=w661) -> (error out=w660:errorcluster)
            n288 = Merge Errors(w660, w656) -> (w655:errorcluster)
          }
          frame "Refresh_Image" {
            w677 = 0.0 ("Z Scale.Range:Minimum")
            # "Call command has to be push to the end not start of the queue."
            n289 = Unbundle By Name(w685) -> ("Para."=w684:variant)
            n290 = Variant To Data(type=1 ("PeakOI #"), Variant=w684) -> (data=w681:i32)  [unwired: 1 in, 1 out]
            n291 = Array Subset(array=w688, index (dim 2)=w681, length (dim 2)=1 ("length")) -> (w687:dbl[][][])  [unwired: 4 in]
            n292 = control-ref of="Intensity Graph"() -> (w680:refnum<vi>)
            n293 = Array Size(array=w687) -> (size(s)=w686:i32[])
            n294 = Index Array(array=w686) -> (element #1=w676:i32, element #2=w675:i32)  [unwired: 3 in, 1 out]
            n295 = Max & Min(x=w676, y=w675) -> (max(x,y)=w674:i32)  [unwired: 1 out]
            n296 = Reshape Array(w687, w676, w675) -> (w679:dbl[][])
            "Intensity Graph" <- w679
            n297 = Array Max & Min(array=w679) -> (max value=w678:dbl)  [unwired: 3 out]
            n298 = property class="IntGraph (strict)"(reference=w680, "ZScale.Maximum"=w678, "ZScale.Minimum"=w677, "XScale.Minimum"=w677, "XScale.Maximum"=w674, "YScale.Minimum"=w677, "YScale.Maximum"=w674) -> ()  [unwired: 1 in, 2 out]
          }
          frame "Save_Image" {
            # "Call command has to be push to the end not start of the queue."
            n299 = control-ref of="Intensity Graph"() -> (w729:refnum<vi>)
            n300 = Unbundle By Name(w735) -> ("Para."=w734:variant)
            n301 = control-ref of="Peaks of Interest"() -> (w702:refnum<vi>)
            n302 = Variant To Data(type=1 ("PeakOI #"), Variant=w734) -> (data=w700:i32)  [unwired: 1 in, 1 out]
            n303 = property class="Tbl (strict)"(reference=w702) -> ("Value"=w701:string[][])  [unwired: 1 in, 2 out]
            n304 = property class="IntGraph (strict)" props=["Color Table", "ZScale", "Maximum", "ZScale", "Minimum", "XScale", "Minimum", "XScale", "Maximum", "YScale", "Minimum", "YScale", "Maximum"](reference=w729) -> ("Color Table"=w706:u32[], "ZScale.Maximum"=w707:dbl, "ZScale.Minimum"=w708:dbl)  [unwired: 1 in, 6 out]
            n305 = control-ref of="Export File Path"() -> (w704:refnum<vi>)
            n306 = Index Array(array=w701, index (row) #1=w700, index (col) #1=0 ("disabled index (col)"), index (row) #2=w700, index (col) #2=1 ("disabled index (col)")) -> (element #1=w697:string, element #2=w696:string)
            n307 = Array Subset(array=w738, index (dim 2)=w700, length (dim 2)=1 ("length")) -> (w737:dbl[][][])  [unwired: 4 in]
            n308 = property class="Path"(reference=w704) -> ("Value"=w703:path)  [unwired: 1 in, 2 out]
            n309 = Array Size(array=w737) -> (size(s)=w736:i32[])
            n310 = Index Array(array=w736) -> (element #1=w731:i32, element #2=w730:i32)  [unwired: 3 in, 1 out]
            n311 = Reshape Array(w737, w731, w730) -> (w705:dbl[][])
            n312 = Strip Path(path=w703) -> (stripped path=w709:path, name=w713:string)
            n313 = Subtract(x=w707, y=w708) -> (x-y=w719:dbl)
            n314 = Subtract(x=w705, y=w708) -> (x-y=w728:dbl[][])
            n315 = xnode "Match Regular Expression"("input string"=w713, "regular expression"="(\\..[^.]*$)") -> ("before match"=w726:string)  [unwired: 4 in, 4 out]
            n316 = Format Into String(format string="_%s(+-%s)", w697, w696) -> (resulting string=w725:string)  [unwired: 2 in, 1 out]
            n317 = Divide(x=256.0 ("Img_coeff."), y=w719) -> (x/y=w721:dbl)
            n318 = Array Size(array=w728) -> (size(s)=w714:i32[])
            n319 = Compound Arithmetic op=MULTIPLY(w721, w728) -> (w722:dbl[][])
            n320 = Transpose 2D Array(2D array=w722) -> (transposed array=w723:dbl[][])
            n321 = Index Array(array=w714) -> (element #1=w716:i32, element #2=w717:i32)  [unwired: 2 in]
            n322 = Concatenate Strings(w726, w725, ".png" ("string")) -> (w710:string)
            n323 = Round Toward -Infinity(1:w723) -> (0:w724:dbl[][])
            n324 = Multiply(x=w716, y=w717) -> (x*y=w718:i32)
            n325 = Build Path(base path=w709, name or relative path=w710) -> (appended path=w711:path)
            n326 = To Unsigned Byte Integer(number=w724) -> (unsigned 8bit integer=w715:u8[][])
            n327 = disable-structure shown="Enabled" {
              disable-tunnel: w706 -> [w756 _]
              disable-tunnel: w711 -> [w755 w759]
              disable-tunnel: w715 -> [w751 w760]
              disable-tunnel: w716 -> [w749 _]
              disable-tunnel: w717 -> [w748 _]
              disable-tunnel: w718 -> [w747 _]
              frame Enabled {
                n328 = Reshape Array(w751, w747) -> (w750:u8[])
                n329 = Bundle By Name(cluster=T24 {"image type"=0, "image depth"=32, "image"=[], "mask"=[], "colors"=[], "Rectangle"={"left"=0, "top"=0, "right"=256, "bottom"=256}} ("Image Data 2"), "colors"=w756, "image type"=0, "image depth"=8, "image"=w750, "Rectangle.right"=w749, "Rectangle.bottom"=w748) -> (w746:T24)
                n330 = call <vilib>:"Write PNG File.vi"("image data"=w746, "path to PNG file"=w755) -> ("error out"=w745:errorcluster)  [unwired: 8 in, 1 out]
                n331 = call <vilib>:"Clear Errors.vi"("error in (no error)"=w745) -> ()  [unwired: 6 in, 1 out]
              }
              frame Disabled {
                n332 = call "IMAQ ArrayToImage"("Image Pixels (U8)"=w760) -> ("Image Out"=w758:T27)  [unwired: 9 in, 1 out]
                n333 = call-poly "IMAQ Write File 2"("TIFF Options"=T25 {"Rows Per Strip"=0, "Photometric"=1, "Compression Type"=3}, "File Path"=w759, "Image"=w758) -> ()  [unwired: 7 in, 2 out]
              }
            }
          }
        }
        n334 = call <userlib>:"ErrorLog.vi"("error in (no error)"=w151) -> ("error out"=w150:errorcluster)  [unwired: 10 in]
      }
      frame Error {
      }
    }
    "Iteration" <- w126
  }
  n335 = Release Queue "Release Queue\nAfter all quit."(queue=w15, error in (no error)=w17) -> (error out=→"error out":errorcluster)  [unwired: 1 in, 2 out]
  n336 = disable-structure "For legacy files, manually add EOL mark" shown="Disabled" {
    frame Disabled {
      w881 = FALSE  # True for missing EOL (Legacy)
      n337 = And(y=w881) -> (x .and. y?=w880:bool)  [unwired: 1 in]
      n338 = case "For Legacy Code" shown="True" w880 {
        tunnel: _ -> [_ w887]
        frame False {
        }
        frame True {
          n339 = Type Cast(type="", x=ProcessStates."EndOfLine") -> (*(type *) &x=w886:string)
          n340 = Bundle By Name(cluster=T18 {"SampleRate"=-1.0, "TrigDelay"=0.0, "SpecLength"=0.0, "DAQ_Range"=0.0, "Average#"=0, "Position"=[], "Spectrum"=[], "Calibr."=[], "Pressure"=-1.0, "Desp_LaserEnergy"=-1.0, "PI_LaserEnergy"=-1.0, "Voltages Table"=[], "ProcMode"=enum."None", "Threshold"=-1.0, "Comment"="", "TickCount"=0.0, "Time Stamp"=timestamp(0 s since 1904-01-01)} ("Value"), "Comment"=w886) -> (w882:T18)
          n341 = Enqueue Element At Opposite End(queue=w887, element=w882) -> ()  [unwired: 2 in, 3 out]
        }
      }
    }
    frame Enabled {
    }
  }
